vi "函数类型3测试.vi"() -> ()   [LabVIEW 2010]
uses:
  全局量/试验配置信息.vi
panel:
  out "合格？":bool[](array[boolean])
  in  "第几组数据":i32
  in  "同步_A2":i32
  in  "同步_A1":i32
  in  "数组_输入值":enum16{"0", "1"}[](array[ring])
  in  "数组_选择?":bool[](array[boolean])
  in  "btn_置1_5":bool
  in  "btn_置1_4":bool
  in  "btn_置1_3":bool
  in  "btn_置1_2":bool
  in  "btn_全选_5":bool
  in  "btn_全选_4":bool
  in  "btn_全选_3":bool
  in  "btn_全选_2":bool
  in  "btn_置1_1":bool
  in  "btn_全选_1":bool
  in  "CAN端口":u16
  out "light_80":bool
  out "light_79":bool
  out "light_78":bool
  out "light_77":bool
  out "light_76":bool
  out "light_75":bool
  out "light_74":bool
  out "light_73":bool
  out "light_72":bool
  out "light_71":bool
  out "light_70":bool
  out "light_69":bool
  out "light_68":bool
  out "light_67":bool
  out "light_66":bool
  out "light_65":bool
  in  "输入值_73":enum16{"0", "1"}(ring)
  in  "输入值_80":enum16{"0", "1"}(ring)
  in  "输入值_79":enum16{"0", "1"}(ring)
  in  "输入值_78":enum16{"0", "1"}(ring)
  in  "输入值_77":enum16{"0", "1"}(ring)
  in  "输入值_76":enum16{"0", "1"}(ring)
  in  "输入值_75":enum16{"0", "1"}(ring)
  in  "输入值_74":enum16{"0", "1"}(ring)
  in  "输入值_65":enum16{"0", "1"}(ring)
  in  "输入值_72":enum16{"0", "1"}(ring)
  in  "输入值_71":enum16{"0", "1"}(ring)
  in  "输入值_70":enum16{"0", "1"}(ring)
  in  "输入值_69":enum16{"0", "1"}(ring)
  in  "输入值_68":enum16{"0", "1"}(ring)
  in  "输入值_67":enum16{"0", "1"}(ring)
  in  "输入值_66":enum16{"0", "1"}(ring)
  in  "单选_第73路":bool
  in  "单选_第80路":bool
  in  "单选_第79路":bool
  in  "单选_第78路":bool
  in  "单选_第77路":bool
  in  "单选_第76路":bool
  in  "单选_第75路":bool
  in  "单选_第74路":bool
  in  "单选_第65路":bool
  in  "单选_第72路":bool
  in  "单选_第71路":bool
  in  "单选_第70路":bool
  in  "单选_第69路":bool
  in  "单选_第68路":bool
  in  "单选_第67路":bool
  in  "单选_第66路":bool
  out "light_64":bool
  out "light_63":bool
  out "light_62":bool
  out "light_61":bool
  out "light_60":bool
  out "light_59":bool
  out "light_58":bool
  out "light_57":bool
  out "light_56":bool
  out "light_55":bool
  out "light_54":bool
  out "light_53":bool
  out "light_52":bool
  out "light_51":bool
  out "light_50":bool
  out "light_49":bool
  in  "输入值_57":enum16{"0", "1"}(ring)
  in  "输入值_64":enum16{"0", "1"}(ring)
  in  "输入值_63":enum16{"0", "1"}(ring)
  in  "输入值_62":enum16{"0", "1"}(ring)
  in  "输入值_61":enum16{"0", "1"}(ring)
  in  "输入值_60":enum16{"0", "1"}(ring)
  in  "输入值_59":enum16{"0", "1"}(ring)
  in  "输入值_58":enum16{"0", "1"}(ring)
  in  "输入值_49":enum16{"0", "1"}(ring)
  in  "输入值_56":enum16{"0", "1"}(ring)
  in  "输入值_55":enum16{"0", "1"}(ring)
  in  "输入值_54":enum16{"0", "1"}(ring)
  in  "输入值_53":enum16{"0", "1"}(ring)
  in  "输入值_52":enum16{"0", "1"}(ring)
  in  "输入值_51":enum16{"0", "1"}(ring)
  in  "输入值_50":enum16{"0", "1"}(ring)
  in  "单选_第57路":bool
  in  "单选_第64路":bool
  in  "单选_第63路":bool
  in  "单选_第62路":bool
  in  "单选_第61路":bool
  in  "单选_第60路":bool
  in  "单选_第59路":bool
  in  "单选_第58路":bool
  in  "单选_第49路":bool
  in  "单选_第56路":bool
  in  "单选_第55路":bool
  in  "单选_第54路":bool
  in  "单选_第53路":bool
  in  "单选_第52路":bool
  in  "单选_第51路":bool
  in  "单选_第50路":bool
  out "light_48":bool
  out "light_47":bool
  out "light_46":bool
  out "light_45":bool
  out "light_44":bool
  out "light_43":bool
  out "light_42":bool
  out "light_41":bool
  out "light_40":bool
  out "light_39":bool
  out "light_38":bool
  out "light_37":bool
  out "light_36":bool
  out "light_35":bool
  out "light_34":bool
  out "light_33":bool
  in  "输入值_41":enum16{"0", "1"}(ring)
  in  "输入值_48":enum16{"0", "1"}(ring)
  in  "输入值_47":enum16{"0", "1"}(ring)
  in  "输入值_46":enum16{"0", "1"}(ring)
  in  "输入值_45":enum16{"0", "1"}(ring)
  in  "输入值_44":enum16{"0", "1"}(ring)
  in  "输入值_43":enum16{"0", "1"}(ring)
  in  "输入值_42":enum16{"0", "1"}(ring)
  in  "输入值_33":enum16{"0", "1"}(ring)
  in  "输入值_40":enum16{"0", "1"}(ring)
  in  "输入值_39":enum16{"0", "1"}(ring)
  in  "输入值_38":enum16{"0", "1"}(ring)
  in  "输入值_37":enum16{"0", "1"}(ring)
  in  "输入值_36":enum16{"0", "1"}(ring)
  in  "输入值_35":enum16{"0", "1"}(ring)
  in  "输入值_34":enum16{"0", "1"}(ring)
  in  "单选_第41路":bool
  in  "单选_第48路":bool
  in  "单选_第47路":bool
  in  "单选_第46路":bool
  in  "单选_第45路":bool
  in  "单选_第44路":bool
  in  "单选_第43路":bool
  in  "单选_第42路":bool
  in  "单选_第33路":bool
  in  "单选_第40路":bool
  in  "单选_第39路":bool
  in  "单选_第38路":bool
  in  "单选_第37路":bool
  in  "单选_第36路":bool
  in  "单选_第35路":bool
  in  "单选_第34路":bool
  out "light_32":bool
  out "light_31":bool
  out "light_30":bool
  out "light_29":bool
  out "light_28":bool
  out "light_27":bool
  out "light_26":bool
  out "light_25":bool
  out "light_24":bool
  out "light_23":bool
  out "light_22":bool
  out "light_21":bool
  out "light_20":bool
  out "light_19":bool
  out "light_18":bool
  out "light_17":bool
  in  "输入值_25":enum16{"0", "1"}(ring)
  in  "输入值_32":enum16{"0", "1"}(ring)
  in  "输入值_31":enum16{"0", "1"}(ring)
  in  "输入值_30":enum16{"0", "1"}(ring)
  in  "输入值_29":enum16{"0", "1"}(ring)
  in  "输入值_28":enum16{"0", "1"}(ring)
  in  "输入值_27":enum16{"0", "1"}(ring)
  in  "输入值_26":enum16{"0", "1"}(ring)
  in  "输入值_17":enum16{"0", "1"}(ring)
  in  "输入值_24":enum16{"0", "1"}(ring)
  in  "输入值_23":enum16{"0", "1"}(ring)
  in  "输入值_22":enum16{"0", "1"}(ring)
  in  "输入值_21":enum16{"0", "1"}(ring)
  in  "输入值_20":enum16{"0", "1"}(ring)
  in  "输入值_19":enum16{"0", "1"}(ring)
  in  "输入值_18":enum16{"0", "1"}(ring)
  in  "单选_第25路":bool
  in  "单选_第32路":bool
  in  "单选_第31路":bool
  in  "单选_第30路":bool
  in  "单选_第29路":bool
  in  "单选_第28路":bool
  in  "单选_第27路":bool
  in  "单选_第26路":bool
  in  "单选_第17路":bool
  in  "单选_第24路":bool
  in  "单选_第23路":bool
  in  "单选_第22路":bool
  in  "单选_第21路":bool
  in  "单选_第20路":bool
  in  "单选_第19路":bool
  in  "单选_第18路":bool
  in  "D_IN_5":string[][](table) caption="表格"
  in  "D_IN_4":string[][](table) caption="表格"
  in  "D_IN_3":string[][](table) caption="表格"
  in  "D_IN_2":string[][](table) caption="表格"
  out "light_16":bool
  out "light_15":bool
  out "light_14":bool
  out "light_13":bool
  out "light_12":bool
  out "light_11":bool
  out "light_10":bool
  out "light_9":bool
  out "light_8":bool
  out "light_7":bool
  out "light_6":bool
  out "light_5":bool
  out "light_4":bool
  out "light_3":bool
  out "light_2":bool
  out "light_1":bool
  in  "输入值_9":enum16{"0", "1"}(ring)
  in  "输入值_16":enum16{"0", "1"}(ring)
  in  "输入值_15":enum16{"0", "1"}(ring)
  in  "输入值_14":enum16{"0", "1"}(ring)
  in  "输入值_13":enum16{"0", "1"}(ring)
  in  "输入值_12":enum16{"0", "1"}(ring)
  in  "输入值_11":enum16{"0", "1"}(ring)
  in  "输入值_10":enum16{"0", "1"}(ring)
  in  "输入值_1":enum16{"0", "1"}(ring)
  in  "输入值_8":enum16{"0", "1"}(ring)
  in  "输入值_7":enum16{"0", "1"}(ring)
  in  "输入值_6":enum16{"0", "1"}(ring)
  in  "输入值_5":enum16{"0", "1"}(ring)
  in  "输入值_4":enum16{"0", "1"}(ring)
  in  "输入值_3":enum16{"0", "1"}(ring)
  in  "输入值_2":enum16{"0", "1"}(ring)
  in  "单选_第9路":bool
  in  "单选_第16路":bool
  in  "单选_第15路":bool
  in  "单选_第14路":bool
  in  "单选_第13路":bool
  in  "单选_第12路":bool
  in  "单选_第11路":bool
  in  "单选_第10路":bool
  in  "单选_第1路":bool
  in  "单选_第8路":bool
  in  "单选_第7路":bool
  in  "单选_第6路":bool
  in  "单选_第5路":bool
  in  "单选_第4路":bool
  in  "单选_第3路":bool
  in  "单选_第2路":bool
  in  "D_IN_1":string[][](table) caption="表格"
  out "关闭？":bool
  out "测试结论":string
  in  "btn_置0":bool
  in  "btn_置1":bool
  in  "btn_反选":bool
  in  "btn_全选":bool
  in  "btn_关闭":bool
  in  "btn_开始试验":bool
  # "第一组数字量测试"
  # "第二组数字量测试"
  # "第三组数字量测试"
  # "第四组数字量测试"
  # "第五组数字量测试"
  # "测试结论："
  # "80"
  # "80"
  # "80"
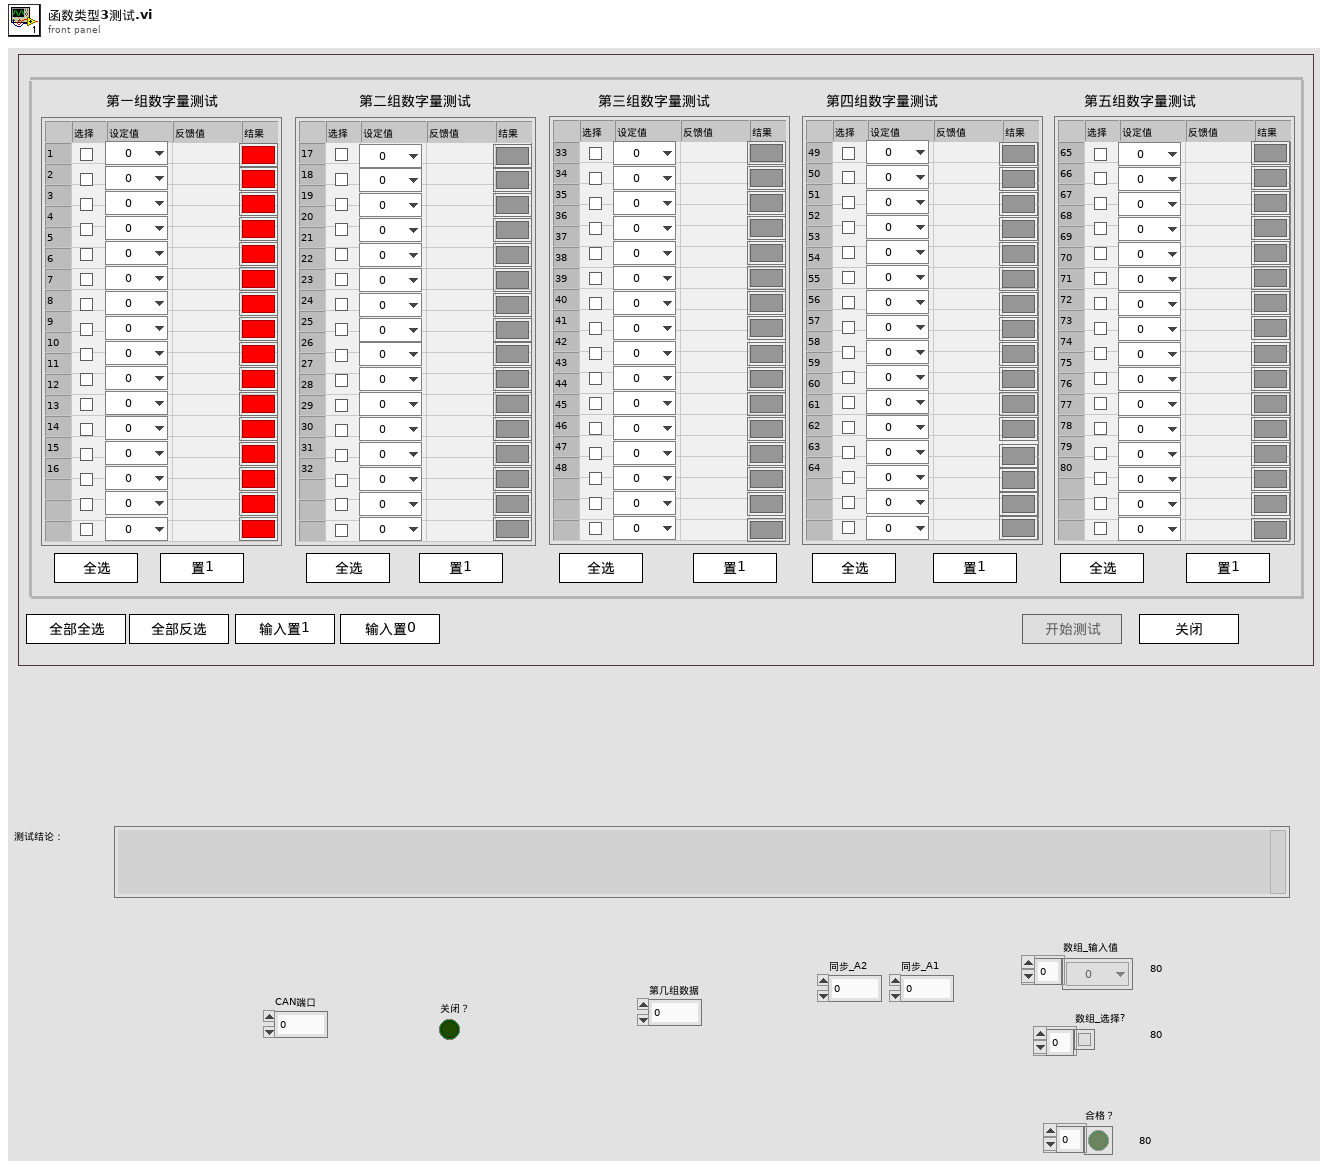
[diagram p1: front panel]
types:
  T1 = enum8{"Enabled", "Disabled", "Disabled and Grayed Out"}
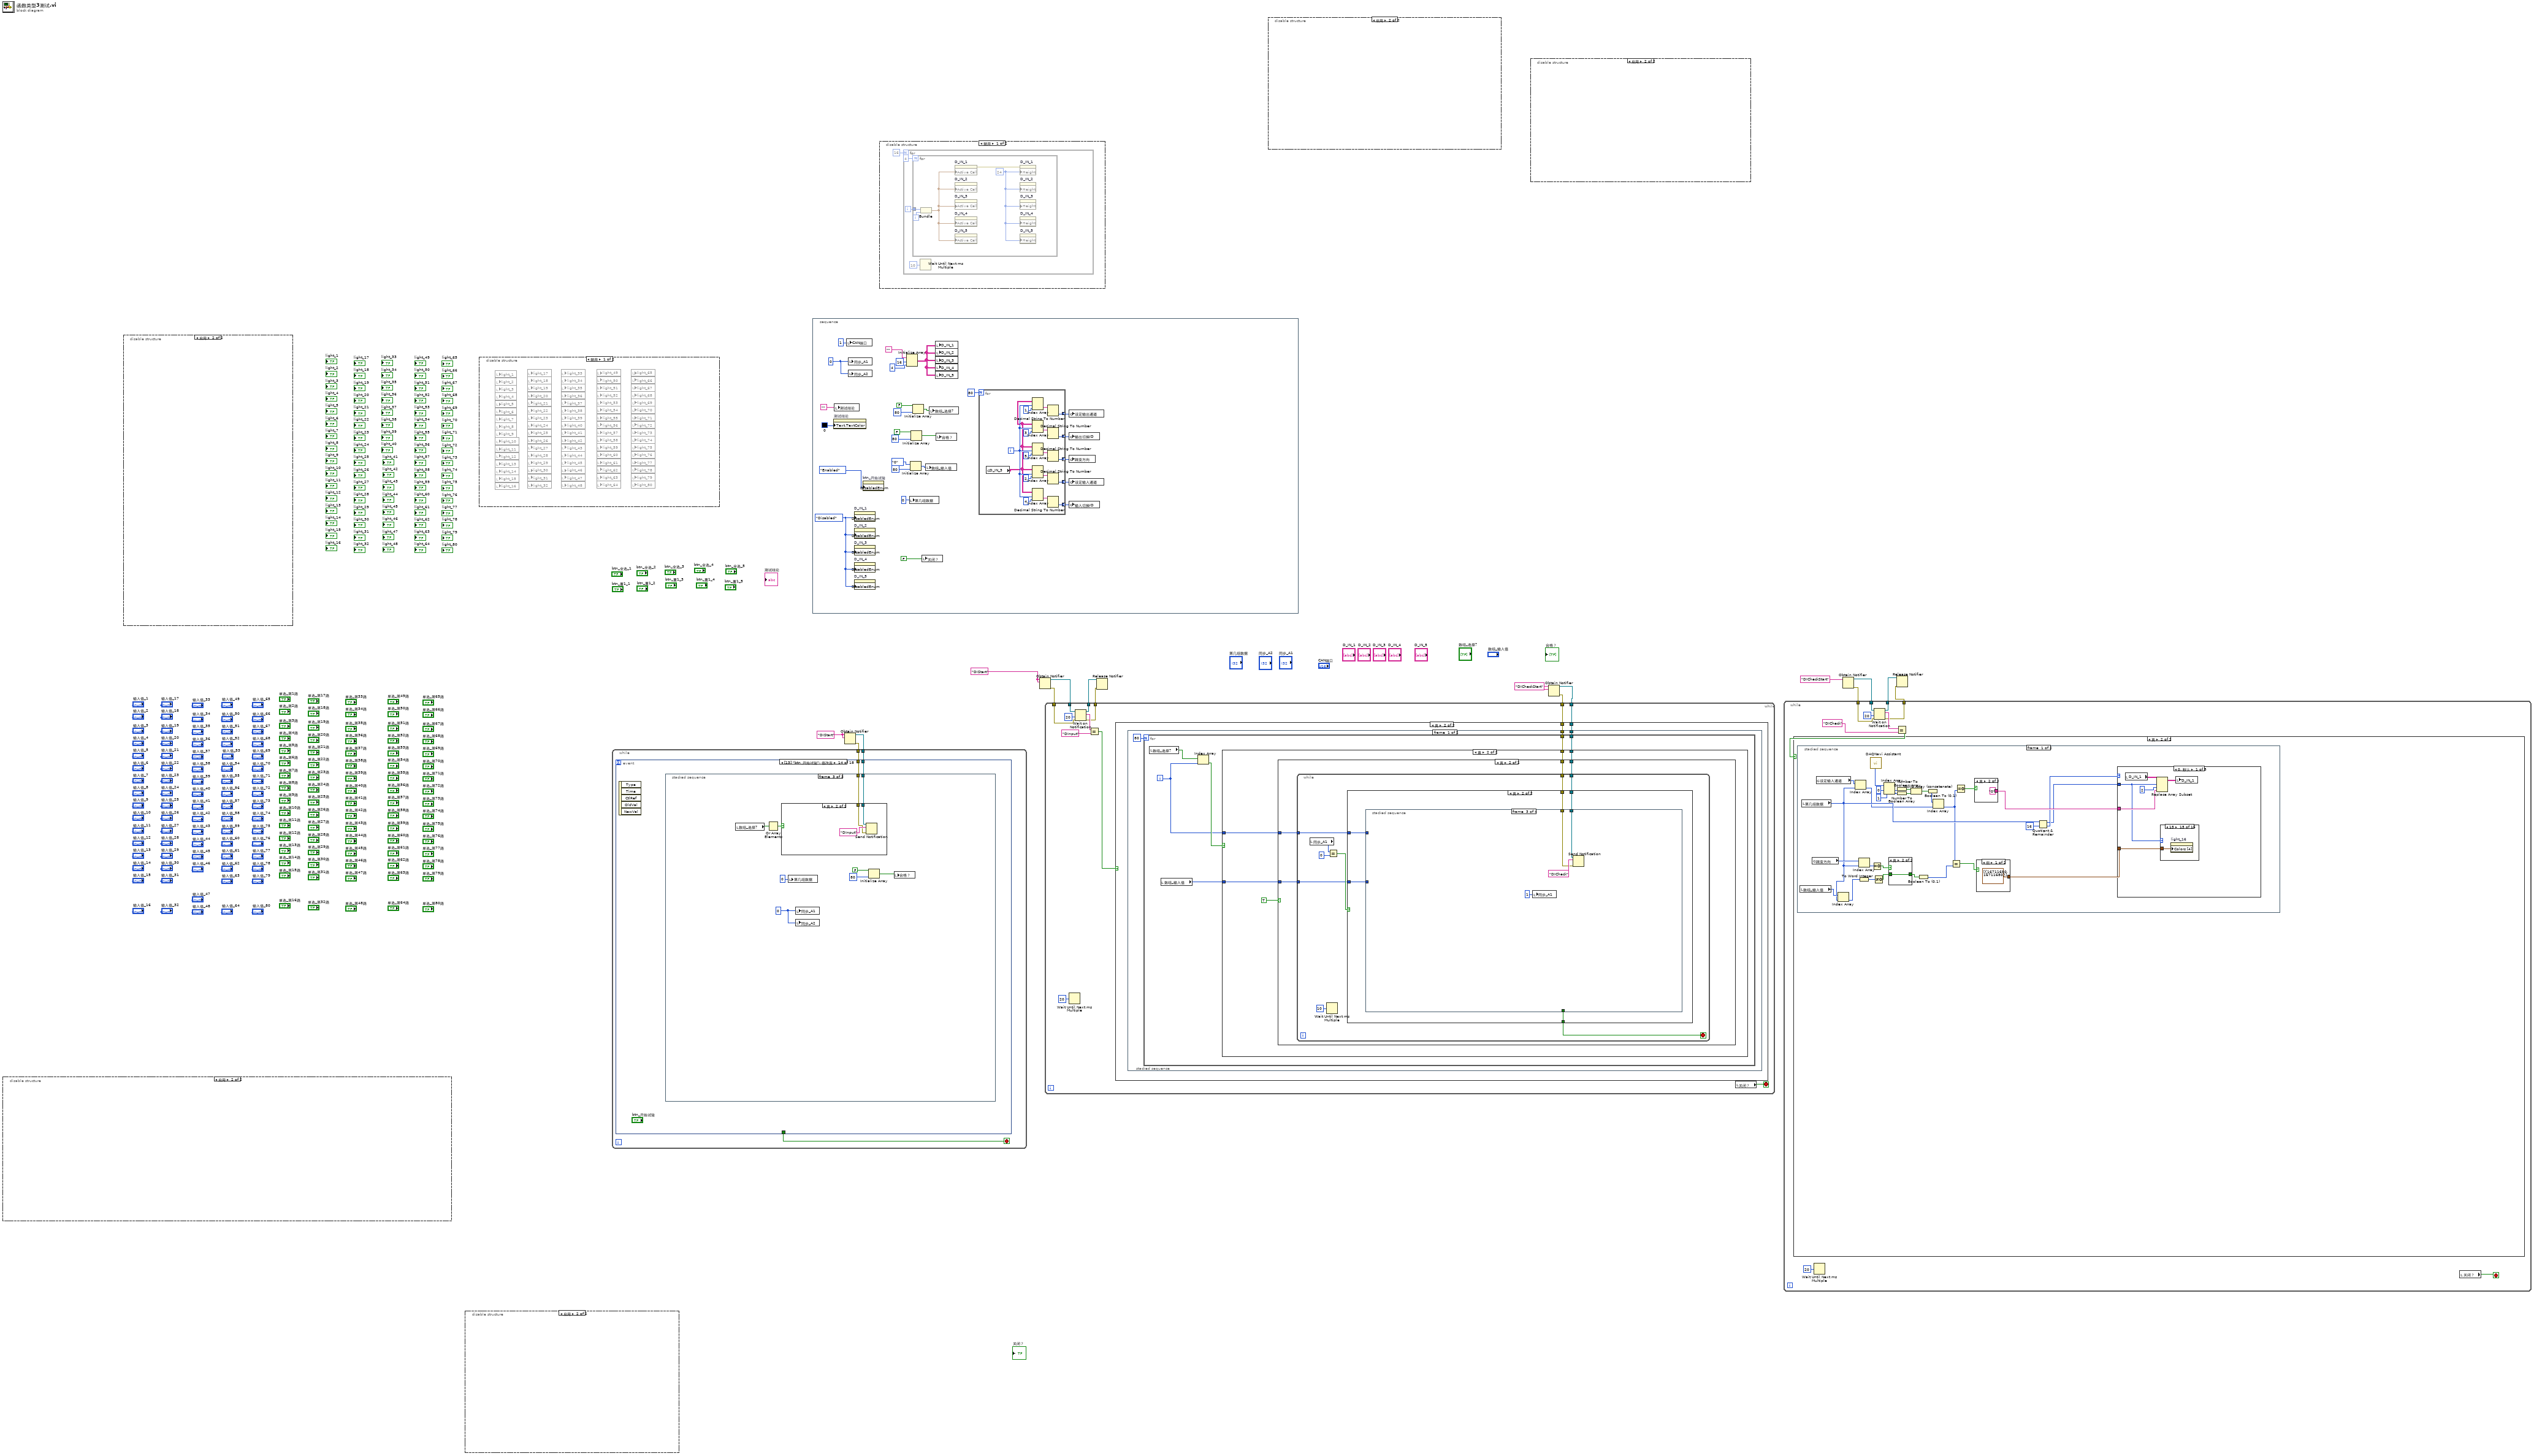
[diagram p0: block diagram]
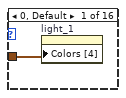
[diagram p4: hidden frame]
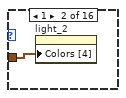
[diagram p5: hidden frame]
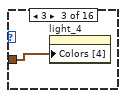
[diagram p6: hidden frame]
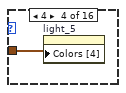
[diagram p7: hidden frame]
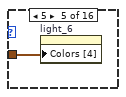
[diagram p8: hidden frame]
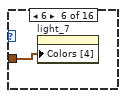
[diagram p9: hidden frame]
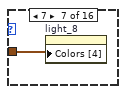
[diagram p10: hidden frame]
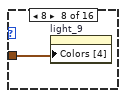
[diagram p11: hidden frame]
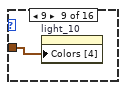
[diagram p12: hidden frame]
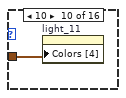
[diagram p13: hidden frame]
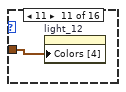
[diagram p14: hidden frame]
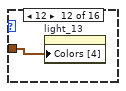
[diagram p15: hidden frame]
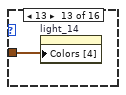
[diagram p16: hidden frame]
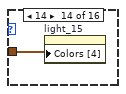
[diagram p17: hidden frame]
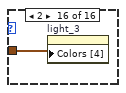
[diagram p18: hidden frame]
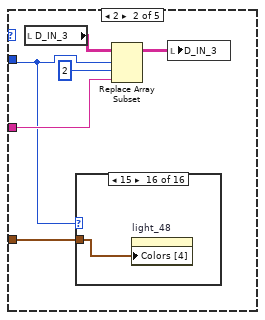
[diagram p19: hidden frame]
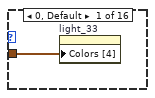
[diagram p20: hidden frame]
diagram:
  w4 = "DICheckStart" ("名称（未命名）")
  w6 = "DIStart" ("名称（未命名）")
  w7 = "DICheckStart" ("名称（未命名）")
  w8 = "DIStart" ("名称（未命名）")
  n1 = disable-structure shown="启用" {
    frame Disabled {
      n2 = local read "单选_第1路"() -> ()  [unwired: 1 in]
      n3 = local read "单选_第2路"() -> ()  [unwired: 1 in]
      n4 = local read "单选_第3路"() -> ()  [unwired: 1 in]
      n5 = local read "单选_第4路"() -> ()  [unwired: 1 in]
      n6 = local read "单选_第5路"() -> ()  [unwired: 1 in]
      n7 = local read "单选_第6路"() -> ()  [unwired: 1 in]
      n8 = local read "单选_第7路"() -> ()  [unwired: 1 in]
      n9 = local read "单选_第8路"() -> ()  [unwired: 1 in]
      n10 = local read "单选_第9路"() -> ()  [unwired: 1 in]
      n11 = local read "单选_第10路"() -> ()  [unwired: 1 in]
      n12 = local read "单选_第11路"() -> ()  [unwired: 1 in]
      n13 = local read "单选_第12路"() -> ()  [unwired: 1 in]
      n14 = local read "单选_第13路"() -> ()  [unwired: 1 in]
      n15 = local read "单选_第14路"() -> ()  [unwired: 1 in]
      n16 = local read "单选_第15路"() -> ()  [unwired: 1 in]
      n17 = local read "单选_第16路"() -> ()  [unwired: 1 in]
      n18 = local read "单选_第17路"() -> ()  [unwired: 1 in]
      n19 = local read "单选_第18路"() -> ()  [unwired: 1 in]
      n20 = local read "单选_第19路"() -> ()  [unwired: 1 in]
      n21 = local read "单选_第20路"() -> ()  [unwired: 1 in]
      n22 = local read "单选_第21路"() -> ()  [unwired: 1 in]
      n23 = local read "单选_第22路"() -> ()  [unwired: 1 in]
      n24 = local read "单选_第23路"() -> ()  [unwired: 1 in]
      n25 = local read "单选_第24路"() -> ()  [unwired: 1 in]
      n26 = local read "单选_第25路"() -> ()  [unwired: 1 in]
      n27 = local read "单选_第26路"() -> ()  [unwired: 1 in]
      n28 = local read "单选_第27路"() -> ()  [unwired: 1 in]
      n29 = local read "单选_第28路"() -> ()  [unwired: 1 in]
      n30 = local read "单选_第29路"() -> ()  [unwired: 1 in]
      n31 = local read "单选_第30路"() -> ()  [unwired: 1 in]
      n32 = local read "单选_第31路"() -> ()  [unwired: 1 in]
      n33 = local read "单选_第32路"() -> ()  [unwired: 1 in]
      n34 = local read "单选_第33路"() -> ()  [unwired: 1 in]
      n35 = local read "单选_第34路"() -> ()  [unwired: 1 in]
      n36 = local read "单选_第35路"() -> ()  [unwired: 1 in]
      n37 = local read "单选_第36路"() -> ()  [unwired: 1 in]
      n38 = local read "单选_第37路"() -> ()  [unwired: 1 in]
      n39 = local read "单选_第38路"() -> ()  [unwired: 1 in]
      n40 = local read "单选_第39路"() -> ()  [unwired: 1 in]
      n41 = local read "单选_第40路"() -> ()  [unwired: 1 in]
      n42 = local read "单选_第41路"() -> ()  [unwired: 1 in]
      n43 = local read "单选_第42路"() -> ()  [unwired: 1 in]
      n44 = local read "单选_第43路"() -> ()  [unwired: 1 in]
      n45 = local read "单选_第44路"() -> ()  [unwired: 1 in]
      n46 = local read "单选_第45路"() -> ()  [unwired: 1 in]
      n47 = local read "单选_第46路"() -> ()  [unwired: 1 in]
      n48 = local read "单选_第47路"() -> ()  [unwired: 1 in]
      n49 = local read "单选_第48路"() -> ()  [unwired: 1 in]
      n50 = local read "单选_第49路"() -> ()  [unwired: 1 in]
      n51 = local read "单选_第50路"() -> ()  [unwired: 1 in]
      n52 = local read "单选_第51路"() -> ()  [unwired: 1 in]
      n53 = local read "单选_第52路"() -> ()  [unwired: 1 in]
      n54 = local read "单选_第53路"() -> ()  [unwired: 1 in]
      n55 = local read "单选_第54路"() -> ()  [unwired: 1 in]
      n56 = local read "单选_第55路"() -> ()  [unwired: 1 in]
      n57 = local read "单选_第56路"() -> ()  [unwired: 1 in]
      n58 = local read "单选_第57路"() -> ()  [unwired: 1 in]
      n59 = local read "单选_第58路"() -> ()  [unwired: 1 in]
      n60 = local read "单选_第59路"() -> ()  [unwired: 1 in]
      n61 = local read "单选_第60路"() -> ()  [unwired: 1 in]
      n62 = local read "单选_第61路"() -> ()  [unwired: 1 in]
      n63 = local read "单选_第62路"() -> ()  [unwired: 1 in]
      n64 = local read "单选_第63路"() -> ()  [unwired: 1 in]
      n65 = local read "单选_第64路"() -> ()  [unwired: 1 in]
      n66 = local read "单选_第71路"() -> ()  [unwired: 1 in]
      n67 = local read "单选_第79路"() -> ()  [unwired: 1 in]
      n68 = local read "单选_第65路"() -> ()  [unwired: 1 in]
      n69 = local read "单选_第66路"() -> ()  [unwired: 1 in]
      n70 = local read "单选_第67路"() -> ()  [unwired: 1 in]
      n71 = local read "单选_第68路"() -> ()  [unwired: 1 in]
      n72 = local read "单选_第69路"() -> ()  [unwired: 1 in]
      n73 = local read "单选_第70路"() -> ()  [unwired: 1 in]
      n74 = local read "单选_第72路"() -> ()  [unwired: 1 in]
      n75 = local read "单选_第73路"() -> ()  [unwired: 1 in]
      n76 = local read "单选_第74路"() -> ()  [unwired: 1 in]
      n77 = local read "单选_第75路"() -> ()  [unwired: 1 in]
      n78 = local read "单选_第76路"() -> ()  [unwired: 1 in]
      n79 = local read "单选_第77路"() -> ()  [unwired: 1 in]
      n80 = local read "单选_第78路"() -> ()  [unwired: 1 in]
      n81 = local read "单选_第80路"() -> ()  [unwired: 1 in]
      n82 = local read "输入值_1"() -> ()  [unwired: 1 in]
      n83 = local read "输入值_2"() -> ()  [unwired: 1 in]
      n84 = local read "输入值_3"() -> ()  [unwired: 1 in]
      n85 = local read "输入值_4"() -> ()  [unwired: 1 in]
      n86 = local read "输入值_5"() -> ()  [unwired: 1 in]
      n87 = local read "输入值_6"() -> ()  [unwired: 1 in]
      n88 = local read "输入值_7"() -> ()  [unwired: 1 in]
      n89 = local read "输入值_8"() -> ()  [unwired: 1 in]
      n90 = local read "输入值_9"() -> ()  [unwired: 1 in]
      n91 = local read "输入值_10"() -> ()  [unwired: 1 in]
      n92 = local read "输入值_11"() -> ()  [unwired: 1 in]
      n93 = local read "输入值_12"() -> ()  [unwired: 1 in]
      n94 = local read "输入值_13"() -> ()  [unwired: 1 in]
      n95 = local read "输入值_14"() -> ()  [unwired: 1 in]
      n96 = local read "输入值_15"() -> ()  [unwired: 1 in]
      n97 = local read "输入值_16"() -> ()  [unwired: 1 in]
      n98 = local read "输入值_17"() -> ()  [unwired: 1 in]
      n99 = local read "输入值_18"() -> ()  [unwired: 1 in]
      n100 = local read "输入值_19"() -> ()  [unwired: 1 in]
      n101 = local read "输入值_20"() -> ()  [unwired: 1 in]
      n102 = local read "输入值_21"() -> ()  [unwired: 1 in]
      n103 = local read "输入值_22"() -> ()  [unwired: 1 in]
      n104 = local read "输入值_23"() -> ()  [unwired: 1 in]
      n105 = local read "输入值_24"() -> ()  [unwired: 1 in]
      n106 = local read "输入值_25"() -> ()  [unwired: 1 in]
      n107 = local read "输入值_26"() -> ()  [unwired: 1 in]
      n108 = local read "输入值_27"() -> ()  [unwired: 1 in]
      n109 = local read "输入值_28"() -> ()  [unwired: 1 in]
      n110 = local read "输入值_29"() -> ()  [unwired: 1 in]
      n111 = local read "输入值_30"() -> ()  [unwired: 1 in]
      n112 = local read "输入值_31"() -> ()  [unwired: 1 in]
      n113 = local read "输入值_32"() -> ()  [unwired: 1 in]
      n114 = local read "输入值_33"() -> ()  [unwired: 1 in]
      n115 = local read "输入值_34"() -> ()  [unwired: 1 in]
      n116 = local read "输入值_35"() -> ()  [unwired: 1 in]
      n117 = local read "输入值_36"() -> ()  [unwired: 1 in]
      n118 = local read "输入值_37"() -> ()  [unwired: 1 in]
      n119 = local read "输入值_38"() -> ()  [unwired: 1 in]
      n120 = local read "输入值_39"() -> ()  [unwired: 1 in]
      n121 = local read "输入值_40"() -> ()  [unwired: 1 in]
      n122 = local read "输入值_41"() -> ()  [unwired: 1 in]
      n123 = local read "输入值_42"() -> ()  [unwired: 1 in]
      n124 = local read "输入值_43"() -> ()  [unwired: 1 in]
      n125 = local read "输入值_44"() -> ()  [unwired: 1 in]
      n126 = local read "输入值_45"() -> ()  [unwired: 1 in]
      n127 = local read "输入值_46"() -> ()  [unwired: 1 in]
      n128 = local read "输入值_47"() -> ()  [unwired: 1 in]
      n129 = local read "输入值_48"() -> ()  [unwired: 1 in]
      n130 = local read "输入值_49"() -> ()  [unwired: 1 in]
      n131 = local read "输入值_50"() -> ()  [unwired: 1 in]
      n132 = local read "输入值_51"() -> ()  [unwired: 1 in]
      n133 = local read "输入值_52"() -> ()  [unwired: 1 in]
      n134 = local read "输入值_53"() -> ()  [unwired: 1 in]
      n135 = local read "输入值_54"() -> ()  [unwired: 1 in]
      n136 = local read "输入值_55"() -> ()  [unwired: 1 in]
      n137 = local read "输入值_56"() -> ()  [unwired: 1 in]
      n138 = local read "输入值_57"() -> ()  [unwired: 1 in]
      n139 = local read "输入值_58"() -> ()  [unwired: 1 in]
      n140 = local read "输入值_59"() -> ()  [unwired: 1 in]
      n141 = local read "输入值_60"() -> ()  [unwired: 1 in]
      n142 = local read "输入值_61"() -> ()  [unwired: 1 in]
      n143 = local read "输入值_62"() -> ()  [unwired: 1 in]
      n144 = local read "输入值_63"() -> ()  [unwired: 1 in]
      n145 = local read "输入值_64"() -> ()  [unwired: 1 in]
      n146 = local read "输入值_65"() -> ()  [unwired: 1 in]
      n147 = local read "输入值_66"() -> ()  [unwired: 1 in]
      n148 = local read "输入值_67"() -> ()  [unwired: 1 in]
      n149 = local read "输入值_68"() -> ()  [unwired: 1 in]
      n150 = local read "输入值_69"() -> ()  [unwired: 1 in]
      n151 = local read "输入值_70"() -> ()  [unwired: 1 in]
      n152 = local read "输入值_71"() -> ()  [unwired: 1 in]
      n153 = local read "输入值_72"() -> ()  [unwired: 1 in]
      n154 = local read "输入值_73"() -> ()  [unwired: 1 in]
      n155 = local read "输入值_74"() -> ()  [unwired: 1 in]
      n156 = local read "输入值_75"() -> ()  [unwired: 1 in]
      n157 = local read "输入值_76"() -> ()  [unwired: 1 in]
      n158 = local read "输入值_77"() -> ()  [unwired: 1 in]
      n159 = local read "输入值_78"() -> ()  [unwired: 1 in]
      n160 = local read "输入值_79"() -> ()  [unwired: 1 in]
      n161 = local read "输入值_80"() -> ()  [unwired: 1 in]
    }
    frame Enabled {
    }
  }
  n162 = disable-structure shown="启用" {
    frame Disabled {
      n163 = property on="light_1" class="Bool (严格)" props=["Colors [4]"]() -> ()  [unwired: 3 in, 2 out]
      n164 = property on="light_2" class="Bool (严格)" props=["Colors [4]"]() -> ()  [unwired: 3 in, 2 out]
      n165 = property on="light_3" class="Bool (严格)" props=["Colors [4]"]() -> ()  [unwired: 3 in, 2 out]
      n166 = property on="light_4" class="Bool (严格)" props=["Colors [4]"]() -> ()  [unwired: 3 in, 2 out]
      n167 = property on="light_5" class="Bool (严格)" props=["Colors [4]"]() -> ()  [unwired: 3 in, 2 out]
      n168 = property on="light_6" class="Bool (严格)" props=["Colors [4]"]() -> ()  [unwired: 3 in, 2 out]
      n169 = property on="light_7" class="Bool (严格)" props=["Colors [4]"]() -> ()  [unwired: 3 in, 2 out]
      n170 = property on="light_8" class="Bool (严格)" props=["Colors [4]"]() -> ()  [unwired: 3 in, 2 out]
      n171 = property on="light_9" class="Bool (严格)" props=["Colors [4]"]() -> ()  [unwired: 3 in, 2 out]
      n172 = property on="light_10" class="Bool (严格)" props=["Colors [4]"]() -> ()  [unwired: 3 in, 2 out]
      n173 = property on="light_11" class="Bool (严格)" props=["Colors [4]"]() -> ()  [unwired: 3 in, 2 out]
      n174 = property on="light_12" class="Bool (严格)" props=["Colors [4]"]() -> ()  [unwired: 3 in, 2 out]
      n175 = property on="light_13" class="Bool (严格)" props=["Colors [4]"]() -> ()  [unwired: 3 in, 2 out]
      n176 = property on="light_14" class="Bool (严格)" props=["Colors [4]"]() -> ()  [unwired: 3 in, 2 out]
      n177 = property on="light_15" class="Bool (严格)" props=["Colors [4]"]() -> ()  [unwired: 3 in, 2 out]
      n178 = property on="light_16" class="Bool (严格)" props=["Colors [4]"]() -> ()  [unwired: 3 in, 2 out]
      n179 = property on="light_17" class="Bool (严格)" props=["Colors [4]"]() -> ()  [unwired: 3 in, 2 out]
      n180 = property on="light_18" class="Bool (严格)" props=["Colors [4]"]() -> ()  [unwired: 3 in, 2 out]
      n181 = property on="light_19" class="Bool (严格)" props=["Colors [4]"]() -> ()  [unwired: 3 in, 2 out]
      n182 = property on="light_20" class="Bool (严格)" props=["Colors [4]"]() -> ()  [unwired: 3 in, 2 out]
      n183 = property on="light_21" class="Bool (严格)" props=["Colors [4]"]() -> ()  [unwired: 3 in, 2 out]
      n184 = property on="light_22" class="Bool (严格)" props=["Colors [4]"]() -> ()  [unwired: 3 in, 2 out]
      n185 = property on="light_23" class="Bool (严格)" props=["Colors [4]"]() -> ()  [unwired: 3 in, 2 out]
      n186 = property on="light_24" class="Bool (严格)" props=["Colors [4]"]() -> ()  [unwired: 3 in, 2 out]
      n187 = property on="light_25" class="Bool (严格)" props=["Colors [4]"]() -> ()  [unwired: 3 in, 2 out]
      n188 = property on="light_26" class="Bool (严格)" props=["Colors [4]"]() -> ()  [unwired: 3 in, 2 out]
      n189 = property on="light_27" class="Bool (严格)" props=["Colors [4]"]() -> ()  [unwired: 3 in, 2 out]
      n190 = property on="light_28" class="Bool (严格)" props=["Colors [4]"]() -> ()  [unwired: 3 in, 2 out]
      n191 = property on="light_29" class="Bool (严格)" props=["Colors [4]"]() -> ()  [unwired: 3 in, 2 out]
      n192 = property on="light_30" class="Bool (严格)" props=["Colors [4]"]() -> ()  [unwired: 3 in, 2 out]
      n193 = property on="light_31" class="Bool (严格)" props=["Colors [4]"]() -> ()  [unwired: 3 in, 2 out]
      n194 = property on="light_32" class="Bool (严格)" props=["Colors [4]"]() -> ()  [unwired: 3 in, 2 out]
      n195 = property on="light_33" class="Bool (严格)" props=["Colors [4]"]() -> ()  [unwired: 3 in, 2 out]
      n196 = property on="light_34" class="Bool (严格)" props=["Colors [4]"]() -> ()  [unwired: 3 in, 2 out]
      n197 = property on="light_35" class="Bool (严格)" props=["Colors [4]"]() -> ()  [unwired: 3 in, 2 out]
      n198 = property on="light_36" class="Bool (严格)" props=["Colors [4]"]() -> ()  [unwired: 3 in, 2 out]
      n199 = property on="light_37" class="Bool (严格)" props=["Colors [4]"]() -> ()  [unwired: 3 in, 2 out]
      n200 = property on="light_38" class="Bool (严格)" props=["Colors [4]"]() -> ()  [unwired: 3 in, 2 out]
      n201 = property on="light_39" class="Bool (严格)" props=["Colors [4]"]() -> ()  [unwired: 3 in, 2 out]
      n202 = property on="light_40" class="Bool (严格)" props=["Colors [4]"]() -> ()  [unwired: 3 in, 2 out]
      n203 = property on="light_41" class="Bool (严格)" props=["Colors [4]"]() -> ()  [unwired: 3 in, 2 out]
      n204 = property on="light_42" class="Bool (严格)" props=["Colors [4]"]() -> ()  [unwired: 3 in, 2 out]
      n205 = property on="light_43" class="Bool (严格)" props=["Colors [4]"]() -> ()  [unwired: 3 in, 2 out]
      n206 = property on="light_44" class="Bool (严格)" props=["Colors [4]"]() -> ()  [unwired: 3 in, 2 out]
      n207 = property on="light_45" class="Bool (严格)" props=["Colors [4]"]() -> ()  [unwired: 3 in, 2 out]
      n208 = property on="light_46" class="Bool (严格)" props=["Colors [4]"]() -> ()  [unwired: 3 in, 2 out]
      n209 = property on="light_47" class="Bool (严格)" props=["Colors [4]"]() -> ()  [unwired: 3 in, 2 out]
      n210 = property on="light_48" class="Bool (严格)" props=["Colors [4]"]() -> ()  [unwired: 3 in, 2 out]
      n211 = property on="light_49" class="Bool (严格)" props=["Colors [4]"]() -> ()  [unwired: 3 in, 2 out]
      n212 = property on="light_50" class="Bool (严格)" props=["Colors [4]"]() -> ()  [unwired: 3 in, 2 out]
      n213 = property on="light_51" class="Bool (严格)" props=["Colors [4]"]() -> ()  [unwired: 3 in, 2 out]
      n214 = property on="light_52" class="Bool (严格)" props=["Colors [4]"]() -> ()  [unwired: 3 in, 2 out]
      n215 = property on="light_53" class="Bool (严格)" props=["Colors [4]"]() -> ()  [unwired: 3 in, 2 out]
      n216 = property on="light_54" class="Bool (严格)" props=["Colors [4]"]() -> ()  [unwired: 3 in, 2 out]
      n217 = property on="light_55" class="Bool (严格)" props=["Colors [4]"]() -> ()  [unwired: 3 in, 2 out]
      n218 = property on="light_56" class="Bool (严格)" props=["Colors [4]"]() -> ()  [unwired: 3 in, 2 out]
      n219 = property on="light_57" class="Bool (严格)" props=["Colors [4]"]() -> ()  [unwired: 3 in, 2 out]
      n220 = property on="light_58" class="Bool (严格)" props=["Colors [4]"]() -> ()  [unwired: 3 in, 2 out]
      n221 = property on="light_59" class="Bool (严格)" props=["Colors [4]"]() -> ()  [unwired: 3 in, 2 out]
      n222 = property on="light_60" class="Bool (严格)" props=["Colors [4]"]() -> ()  [unwired: 3 in, 2 out]
      n223 = property on="light_61" class="Bool (严格)" props=["Colors [4]"]() -> ()  [unwired: 3 in, 2 out]
      n224 = property on="light_62" class="Bool (严格)" props=["Colors [4]"]() -> ()  [unwired: 3 in, 2 out]
      n225 = property on="light_63" class="Bool (严格)" props=["Colors [4]"]() -> ()  [unwired: 3 in, 2 out]
      n226 = property on="light_64" class="Bool (严格)" props=["Colors [4]"]() -> ()  [unwired: 3 in, 2 out]
      n227 = property on="light_65" class="Bool (严格)" props=["Colors [4]"]() -> ()  [unwired: 3 in, 2 out]
      n228 = property on="light_66" class="Bool (严格)" props=["Colors [4]"]() -> ()  [unwired: 3 in, 2 out]
      n229 = property on="light_67" class="Bool (严格)" props=["Colors [4]"]() -> ()  [unwired: 3 in, 2 out]
      n230 = property on="light_68" class="Bool (严格)" props=["Colors [4]"]() -> ()  [unwired: 3 in, 2 out]
      n231 = property on="light_69" class="Bool (严格)" props=["Colors [4]"]() -> ()  [unwired: 3 in, 2 out]
      n232 = property on="light_70" class="Bool (严格)" props=["Colors [4]"]() -> ()  [unwired: 3 in, 2 out]
      n233 = property on="light_71" class="Bool (严格)" props=["Colors [4]"]() -> ()  [unwired: 3 in, 2 out]
      n234 = property on="light_72" class="Bool (严格)" props=["Colors [4]"]() -> ()  [unwired: 3 in, 2 out]
      n235 = property on="light_73" class="Bool (严格)" props=["Colors [4]"]() -> ()  [unwired: 3 in, 2 out]
      n236 = property on="light_74" class="Bool (严格)" props=["Colors [4]"]() -> ()  [unwired: 3 in, 2 out]
      n237 = property on="light_75" class="Bool (严格)" props=["Colors [4]"]() -> ()  [unwired: 3 in, 2 out]
      n238 = property on="light_76" class="Bool (严格)" props=["Colors [4]"]() -> ()  [unwired: 3 in, 2 out]
      n239 = property on="light_77" class="Bool (严格)" props=["Colors [4]"]() -> ()  [unwired: 3 in, 2 out]
      n240 = property on="light_78" class="Bool (严格)" props=["Colors [4]"]() -> ()  [unwired: 3 in, 2 out]
      n241 = property on="light_79" class="Bool (严格)" props=["Colors [4]"]() -> ()  [unwired: 3 in, 2 out]
      n242 = property on="light_80" class="Bool (严格)" props=["Colors [4]"]() -> ()  [unwired: 3 in, 2 out]
    }
    frame Enabled {
    }
  }
  n243 = disable-structure shown="启用" {
    frame Disabled {
      n244 = local read "输入值_1"() -> ()  [unwired: 1 out]
      n245 = local read "输入值_2"() -> ()  [unwired: 1 out]
      n246 = local read "输入值_3"() -> ()  [unwired: 1 out]
      n247 = local read "输入值_4"() -> ()  [unwired: 1 out]
      n248 = local read "输入值_5"() -> ()  [unwired: 1 out]
      n249 = local read "输入值_6"() -> ()  [unwired: 1 out]
      n250 = local read "输入值_7"() -> ()  [unwired: 1 out]
      n251 = local read "输入值_8"() -> ()  [unwired: 1 out]
      n252 = local read "输入值_9"() -> ()  [unwired: 1 out]
      n253 = local read "输入值_10"() -> ()  [unwired: 1 out]
      n254 = local read "输入值_11"() -> ()  [unwired: 1 out]
      n255 = local read "输入值_12"() -> ()  [unwired: 1 out]
      n256 = local read "输入值_13"() -> ()  [unwired: 1 out]
      n257 = local read "输入值_14"() -> ()  [unwired: 1 out]
      n258 = local read "输入值_15"() -> ()  [unwired: 1 out]
      n259 = local read "输入值_16"() -> ()  [unwired: 1 out]
      n260 = local read "输入值_17"() -> ()  [unwired: 1 out]
      n261 = local read "输入值_18"() -> ()  [unwired: 1 out]
      n262 = local read "输入值_19"() -> ()  [unwired: 1 out]
      n263 = local read "输入值_20"() -> ()  [unwired: 1 out]
      n264 = local read "输入值_21"() -> ()  [unwired: 1 out]
      n265 = local read "输入值_22"() -> ()  [unwired: 1 out]
      n266 = local read "输入值_23"() -> ()  [unwired: 1 out]
      n267 = local read "输入值_24"() -> ()  [unwired: 1 out]
      n268 = local read "输入值_25"() -> ()  [unwired: 1 out]
      n269 = local read "输入值_26"() -> ()  [unwired: 1 out]
      n270 = local read "输入值_27"() -> ()  [unwired: 1 out]
      n271 = local read "输入值_28"() -> ()  [unwired: 1 out]
      n272 = local read "输入值_29"() -> ()  [unwired: 1 out]
      n273 = local read "输入值_30"() -> ()  [unwired: 1 out]
      n274 = local read "输入值_31"() -> ()  [unwired: 1 out]
      n275 = local read "输入值_32"() -> ()  [unwired: 1 out]
      n276 = local read "输入值_33"() -> ()  [unwired: 1 out]
      n277 = local read "输入值_34"() -> ()  [unwired: 1 out]
      n278 = local read "输入值_35"() -> ()  [unwired: 1 out]
      n279 = local read "输入值_36"() -> ()  [unwired: 1 out]
      n280 = local read "输入值_37"() -> ()  [unwired: 1 out]
      n281 = local read "输入值_38"() -> ()  [unwired: 1 out]
      n282 = local read "输入值_39"() -> ()  [unwired: 1 out]
      n283 = local read "输入值_40"() -> ()  [unwired: 1 out]
      n284 = local read "输入值_41"() -> ()  [unwired: 1 out]
      n285 = local read "输入值_42"() -> ()  [unwired: 1 out]
      n286 = local read "输入值_43"() -> ()  [unwired: 1 out]
      n287 = local read "输入值_44"() -> ()  [unwired: 1 out]
      n288 = local read "输入值_45"() -> ()  [unwired: 1 out]
      n289 = local read "输入值_46"() -> ()  [unwired: 1 out]
      n290 = local read "输入值_47"() -> ()  [unwired: 1 out]
      n291 = local read "输入值_48"() -> ()  [unwired: 1 out]
      n292 = local read "输入值_49"() -> ()  [unwired: 1 out]
      n293 = local read "输入值_50"() -> ()  [unwired: 1 out]
      n294 = local read "输入值_51"() -> ()  [unwired: 1 out]
      n295 = local read "输入值_52"() -> ()  [unwired: 1 out]
      n296 = local read "输入值_53"() -> ()  [unwired: 1 out]
      n297 = local read "输入值_54"() -> ()  [unwired: 1 out]
      n298 = local read "输入值_55"() -> ()  [unwired: 1 out]
      n299 = local read "输入值_56"() -> ()  [unwired: 1 out]
      n300 = local read "输入值_57"() -> ()  [unwired: 1 out]
      n301 = local read "输入值_58"() -> ()  [unwired: 1 out]
      n302 = local read "输入值_59"() -> ()  [unwired: 1 out]
      n303 = local read "输入值_60"() -> ()  [unwired: 1 out]
      n304 = local read "输入值_61"() -> ()  [unwired: 1 out]
      n305 = local read "输入值_62"() -> ()  [unwired: 1 out]
      n306 = local read "输入值_63"() -> ()  [unwired: 1 out]
      n307 = local read "输入值_64"() -> ()  [unwired: 1 out]
      n308 = local read "输入值_65"() -> ()  [unwired: 1 out]
      n309 = local read "输入值_66"() -> ()  [unwired: 1 out]
      n310 = local read "输入值_67"() -> ()  [unwired: 1 out]
      n311 = local read "输入值_68"() -> ()  [unwired: 1 out]
      n312 = local read "输入值_69"() -> ()  [unwired: 1 out]
      n313 = local read "输入值_70"() -> ()  [unwired: 1 out]
      n314 = local read "输入值_71"() -> ()  [unwired: 1 out]
      n315 = local read "输入值_72"() -> ()  [unwired: 1 out]
      n316 = local read "输入值_73"() -> ()  [unwired: 1 out]
      n317 = local read "输入值_74"() -> ()  [unwired: 1 out]
      n318 = local read "输入值_75"() -> ()  [unwired: 1 out]
      n319 = local read "输入值_76"() -> ()  [unwired: 1 out]
      n320 = local read "输入值_77"() -> ()  [unwired: 1 out]
      n321 = local read "输入值_78"() -> ()  [unwired: 1 out]
      n322 = local read "输入值_79"() -> ()  [unwired: 1 out]
      n323 = local read "输入值_80"() -> ()  [unwired: 1 out]
    }
    frame Enabled {
    }
  }
  n324 = disable-structure shown="禁用" {
    frame Disabled {
      n325 = local read "light_1"() -> ()  [unwired: 1 in]
      n326 = local read "light_2"() -> ()  [unwired: 1 in]
      n327 = local read "light_3"() -> ()  [unwired: 1 in]
      n328 = local read "light_4"() -> ()  [unwired: 1 in]
      n329 = local read "light_5"() -> ()  [unwired: 1 in]
      n330 = local read "light_6"() -> ()  [unwired: 1 in]
      n331 = local read "light_7"() -> ()  [unwired: 1 in]
      n332 = local read "light_8"() -> ()  [unwired: 1 in]
      n333 = local read "light_9"() -> ()  [unwired: 1 in]
      n334 = local read "light_10"() -> ()  [unwired: 1 in]
      n335 = local read "light_11"() -> ()  [unwired: 1 in]
      n336 = local read "light_12"() -> ()  [unwired: 1 in]
      n337 = local read "light_13"() -> ()  [unwired: 1 in]
      n338 = local read "light_14"() -> ()  [unwired: 1 in]
      n339 = local read "light_15"() -> ()  [unwired: 1 in]
      n340 = local read "light_16"() -> ()  [unwired: 1 in]
      n341 = local read "light_17"() -> ()  [unwired: 1 in]
      n342 = local read "light_18"() -> ()  [unwired: 1 in]
      n343 = local read "light_19"() -> ()  [unwired: 1 in]
      n344 = local read "light_20"() -> ()  [unwired: 1 in]
      n345 = local read "light_21"() -> ()  [unwired: 1 in]
      n346 = local read "light_22"() -> ()  [unwired: 1 in]
      n347 = local read "light_23"() -> ()  [unwired: 1 in]
      n348 = local read "light_24"() -> ()  [unwired: 1 in]
      n349 = local read "light_25"() -> ()  [unwired: 1 in]
      n350 = local read "light_26"() -> ()  [unwired: 1 in]
      n351 = local read "light_27"() -> ()  [unwired: 1 in]
      n352 = local read "light_28"() -> ()  [unwired: 1 in]
      n353 = local read "light_29"() -> ()  [unwired: 1 in]
      n354 = local read "light_30"() -> ()  [unwired: 1 in]
      n355 = local read "light_31"() -> ()  [unwired: 1 in]
      n356 = local read "light_32"() -> ()  [unwired: 1 in]
      n357 = local read "light_33"() -> ()  [unwired: 1 in]
      n358 = local read "light_34"() -> ()  [unwired: 1 in]
      n359 = local read "light_35"() -> ()  [unwired: 1 in]
      n360 = local read "light_36"() -> ()  [unwired: 1 in]
      n361 = local read "light_37"() -> ()  [unwired: 1 in]
      n362 = local read "light_38"() -> ()  [unwired: 1 in]
      n363 = local read "light_39"() -> ()  [unwired: 1 in]
      n364 = local read "light_40"() -> ()  [unwired: 1 in]
      n365 = local read "light_41"() -> ()  [unwired: 1 in]
      n366 = local read "light_42"() -> ()  [unwired: 1 in]
      n367 = local read "light_43"() -> ()  [unwired: 1 in]
      n368 = local read "light_44"() -> ()  [unwired: 1 in]
      n369 = local read "light_45"() -> ()  [unwired: 1 in]
      n370 = local read "light_46"() -> ()  [unwired: 1 in]
      n371 = local read "light_47"() -> ()  [unwired: 1 in]
      n372 = local read "light_48"() -> ()  [unwired: 1 in]
      n373 = local read "light_49"() -> ()  [unwired: 1 in]
      n374 = local read "light_50"() -> ()  [unwired: 1 in]
      n375 = local read "light_51"() -> ()  [unwired: 1 in]
      n376 = local read "light_52"() -> ()  [unwired: 1 in]
      n377 = local read "light_53"() -> ()  [unwired: 1 in]
      n378 = local read "light_54"() -> ()  [unwired: 1 in]
      n379 = local read "light_55"() -> ()  [unwired: 1 in]
      n380 = local read "light_56"() -> ()  [unwired: 1 in]
      n381 = local read "light_57"() -> ()  [unwired: 1 in]
      n382 = local read "light_58"() -> ()  [unwired: 1 in]
      n383 = local read "light_59"() -> ()  [unwired: 1 in]
      n384 = local read "light_60"() -> ()  [unwired: 1 in]
      n385 = local read "light_61"() -> ()  [unwired: 1 in]
      n386 = local read "light_62"() -> ()  [unwired: 1 in]
      n387 = local read "light_63"() -> ()  [unwired: 1 in]
      n388 = local read "light_64"() -> ()  [unwired: 1 in]
      n389 = local read "light_65"() -> ()  [unwired: 1 in]
      n390 = local read "light_66"() -> ()  [unwired: 1 in]
      n391 = local read "light_67"() -> ()  [unwired: 1 in]
      n392 = local read "light_68"() -> ()  [unwired: 1 in]
      n393 = local read "light_69"() -> ()  [unwired: 1 in]
      n394 = local read "light_70"() -> ()  [unwired: 1 in]
      n395 = local read "light_71"() -> ()  [unwired: 1 in]
      n396 = local read "light_72"() -> ()  [unwired: 1 in]
      n397 = local read "light_73"() -> ()  [unwired: 1 in]
      n398 = local read "light_74"() -> ()  [unwired: 1 in]
      n399 = local read "light_75"() -> ()  [unwired: 1 in]
      n400 = local read "light_76"() -> ()  [unwired: 1 in]
      n401 = local read "light_77"() -> ()  [unwired: 1 in]
      n402 = local read "light_78"() -> ()  [unwired: 1 in]
      n403 = local read "light_79"() -> ()  [unwired: 1 in]
      n404 = local read "light_80"() -> ()  [unwired: 1 in]
    }
    frame Enabled {
    }
  }
  n405 = stacked-sequence {
    frame #0 {
      w31 = 0 ("同步_A1")
      w41 = T1."Disabled" ("禁用")
      n406 = property on="测试结论" class="Str"("Text.TextColor"=u32 0) -> ()  [unwired: 2 in, 2 out]
      n407 = local write "测试结论"("") -> ()
      n408 = local write "CAN端口"(u16 1 ("CAN端口")) -> ()
      n409 = local write "同步_A1"(w31) -> ()
      n410 = local write "同步_A2"(w31) -> ()
      n411 = property on="D_IN_1" class="Tbl (严格)"("DisabledEnum"=w41) -> ()  [unwired: 2 in, 2 out]
      n412 = property on="D_IN_2" class="Tbl (严格)"("DisabledEnum"=w41) -> ()  [unwired: 2 in, 2 out]
      n413 = property on="D_IN_3" class="Tbl (严格)"("DisabledEnum"=w41) -> ()  [unwired: 2 in, 2 out]
      n414 = property on="D_IN_4" class="Tbl (严格)"("DisabledEnum"=w41) -> ()  [unwired: 2 in, 2 out]
      n415 = property on="D_IN_5" class="Tbl (严格)"("DisabledEnum"=w41) -> ()  [unwired: 2 in, 2 out]
      n416 = property on="btn_开始试验" class="Bool"("DisabledEnum"=T1."Enabled" ("禁用")) -> ()  [unwired: 2 in, 2 out]
      n417 = Initialize Array("", 16 ("维数大小"), 4 ("维数大小")) -> (w37:string[][])
      n418 = local write "第几组数据"(0 ("第几组数据")) -> ()
      n419 = Initialize Array(enum16{"0", "1"}."0" ("输入值_32"), 80 ("维数大小")) -> (w28:enum16{"0", "1"}[])
      n420 = Initialize Array(FALSE, 80 ("维数大小")) -> (w24:bool[])
      n421 = Initialize Array(FALSE, 80 ("维数大小")) -> (w27:bool[])
      n422 = local write "关闭？"(FALSE) -> ()
      n423 = local write "数组_输入值"(w28) -> ()
      n424 = local write "数组_选择?"(w27) -> ()
      n425 = local write "D_IN_1"(w37) -> ()
      n426 = local write "D_IN_2"(w37) -> ()
      n427 = local write "D_IN_3"(w37) -> ()
      n428 = local write "D_IN_4"(w37) -> ()
      n429 = local write "D_IN_5"(w37) -> ()
      n430 = local write "合格？"(w24) -> ()
      n431 = for {
        N: 80 -> [_]
        tunnel: [w58] -> w22 mode=indexing
        tunnel: [w55] -> w21 mode=indexing
        tunnel: [w52] -> w20 mode=indexing
        tunnel: [w49] -> w19 mode=indexing
        tunnel: [w45] -> w18 mode=indexing
        i -> [w47]
        n432 = global read "试验配置信息.vi" "D_IN_3"() -> (w44:string[][])
        n433 = Index Array(array=w44, index (row)=w47, index (col)=1 ("禁用的索引 (列)")) -> (element=w57:string)
        n434 = Index Array(array=w44, index (row)=w47, index (col)=3 ("禁用的索引 (列)")) -> (element=w53:string)
        n435 = Index Array(array=w44, index (row)=w47, index (col)=5 ("禁用的索引 (列)")) -> (element=w46:string)
        n436 = Index Array(array=w44, index (row)=w47, index (col)=2 ("禁用的索引 (列)")) -> (element=w59:string)
        n437 = Index Array(array=w44, index (row)=w47, index (col)=4 ("禁用的索引 (列)")) -> (element=w50:string)
        n438 = Decimal String To Number(string=w57) -> (number=w55:i32)  [unwired: 2 in, 1 out]
        n439 = Decimal String To Number(string=w53) -> (number=w52:i32)  [unwired: 2 in, 1 out]
        n440 = Decimal String To Number(string=w46) -> (number=w45:i32)  [unwired: 2 in, 1 out]
        n441 = Decimal String To Number(string=w59) -> (number=w58:i32)  [unwired: 2 in, 1 out]
        n442 = Decimal String To Number(string=w50) -> (number=w49:i32)  [unwired: 2 in, 1 out]
      }
      n443 = global write "试验配置信息.vi" "设定输出通道"(w21) -> ()
      n444 = global write "试验配置信息.vi" "输出切换ID"(w20) -> ()
      n445 = global write "试验配置信息.vi" "跳变方向"(w18) -> ()
      n446 = global write "试验配置信息.vi" "设定输入通道"(w22) -> ()
      n447 = global write "试验配置信息.vi" "输入切换ID"(w19) -> ()
    }
  }
  n448 = Obtain Notifier(name (unnamed)=w6, notification data type=w6) -> (notifier out=w5:refnum<notifier>, error out=w1:errorcluster)  [unwired: 2 in, 1 out]
  n449 = while {
    tunnel: w5 -> [w62]
    tunnel: w1 -> [w61]
    stop <- w63 stop-if-true
    n450 = event shown="[13] \"btn_开始试验\": 值改变" {
      selector: _ -> [_ _ _ _ _ _ _ _ _ _ _ _ _ _ _ _ _ _]
      dyn-events: _ -> [_ _ _ _ _ _ _ _ _ _ _ _ _ _ _ _ _ _]
      timeout: _ -> [_ _ _ _ _ _ _ _ _ _ _ _ _ _ _ _ _ _]
      tunnel: [_ w64 w65 _ _ _ _ _ _ _ _ _ _ _ _ _ _ _] -> w63
      tunnel: w62 -> [_ _ _ _ _ _ _ _ _ _ _ _ _ w107 _ _ _ _]
      tunnel: w61 -> [_ _ _ _ _ _ _ _ _ _ _ _ _ w106 _ _ _ _]
      event Timeout {
        n451 = event-data() -> ()  [unwired: 1 in, 2 out]
      }
      event Panel Close {
        w64 = TRUE ("关闭？")
        n452 = event-data() -> ()  [unwired: 1 in, 3 out]
        n453 = local write "关闭？"(w64) -> ()
      }
      event "btn_关闭": Value Change {
        w65 = TRUE
        n454 = event-data() -> ()  [unwired: 1 in, 5 out]
        n455 = local write "关闭？"(w65) -> ()
      }
      event "btn_全选_1": Value Change {
        n456 = event-data() -> ("NewVal"=w67:bool)  [unwired: 1 in, 4 out]
        n457 = case shown="假" w67 {
          tunnel: [FALSE ("单选_第41路") TRUE ("单选_第41路")] -> w66
          frame False {
          }
          frame True {
          }
        }
        n458 = local write "单选_第1路"(w66) -> ()
        n459 = local write "单选_第2路"(w66) -> ()
        n460 = local write "单选_第3路"(w66) -> ()
        n461 = local write "单选_第4路"(w66) -> ()
        n462 = local write "单选_第5路"(w66) -> ()
        n463 = local write "单选_第6路"(w66) -> ()
        n464 = local write "单选_第7路"(w66) -> ()
        n465 = local write "单选_第8路"(w66) -> ()
        n466 = local write "单选_第9路"(w66) -> ()
        n467 = local write "单选_第10路"(w66) -> ()
        n468 = local write "单选_第11路"(w66) -> ()
        n469 = local write "单选_第12路"(w66) -> ()
        n470 = local write "单选_第13路"(w66) -> ()
        n471 = local write "单选_第14路"(w66) -> ()
        n472 = local write "单选_第15路"(w66) -> ()
        n473 = local write "单选_第16路"(w66) -> ()
      }
      event "btn_全选_2": Value Change {
        n474 = event-data() -> ("NewVal"=w71:bool)  [unwired: 1 in, 4 out]
        n475 = case shown="假" w71 {
          tunnel: [FALSE ("单选_第41路") TRUE ("单选_第41路")] -> w70
          frame False {
          }
          frame True {
          }
        }
        n476 = local write "单选_第17路"(w70) -> ()
        n477 = local write "单选_第18路"(w70) -> ()
        n478 = local write "单选_第19路"(w70) -> ()
        n479 = local write "单选_第20路"(w70) -> ()
        n480 = local write "单选_第21路"(w70) -> ()
        n481 = local write "单选_第22路"(w70) -> ()
        n482 = local write "单选_第23路"(w70) -> ()
        n483 = local write "单选_第24路"(w70) -> ()
        n484 = local write "单选_第25路"(w70) -> ()
        n485 = local write "单选_第26路"(w70) -> ()
        n486 = local write "单选_第27路"(w70) -> ()
        n487 = local write "单选_第28路"(w70) -> ()
        n488 = local write "单选_第29路"(w70) -> ()
        n489 = local write "单选_第30路"(w70) -> ()
        n490 = local write "单选_第31路"(w70) -> ()
        n491 = local write "单选_第32路"(w70) -> ()
      }
      event "btn_全选_3": Value Change {
        n492 = event-data() -> ("NewVal"=w75:bool)  [unwired: 1 in, 4 out]
        n493 = case shown="假" w75 {
          tunnel: [FALSE ("单选_第41路") TRUE ("单选_第41路")] -> w74
          frame False {
          }
          frame True {
          }
        }
        n494 = local write "单选_第33路"(w74) -> ()
        n495 = local write "单选_第34路"(w74) -> ()
        n496 = local write "单选_第35路"(w74) -> ()
        n497 = local write "单选_第36路"(w74) -> ()
        n498 = local write "单选_第37路"(w74) -> ()
        n499 = local write "单选_第38路"(w74) -> ()
        n500 = local write "单选_第39路"(w74) -> ()
        n501 = local write "单选_第40路"(w74) -> ()
        n502 = local write "单选_第41路"(w74) -> ()
        n503 = local write "单选_第42路"(w74) -> ()
        n504 = local write "单选_第43路"(w74) -> ()
        n505 = local write "单选_第44路"(w74) -> ()
        n506 = local write "单选_第45路"(w74) -> ()
        n507 = local write "单选_第46路"(w74) -> ()
        n508 = local write "单选_第47路"(w74) -> ()
        n509 = local write "单选_第48路"(w74) -> ()
      }
      event "btn_全选_4": Value Change {
        n510 = event-data() -> ("NewVal"=w79:bool)  [unwired: 1 in, 4 out]
        n511 = case shown="假" w79 {
          tunnel: [FALSE ("单选_第41路") TRUE ("单选_第41路")] -> w78
          frame False {
          }
          frame True {
          }
        }
        n512 = local write "单选_第49路"(w78) -> ()
        n513 = local write "单选_第50路"(w78) -> ()
        n514 = local write "单选_第51路"(w78) -> ()
        n515 = local write "单选_第52路"(w78) -> ()
        n516 = local write "单选_第53路"(w78) -> ()
        n517 = local write "单选_第54路"(w78) -> ()
        n518 = local write "单选_第55路"(w78) -> ()
        n519 = local write "单选_第56路"(w78) -> ()
        n520 = local write "单选_第57路"(w78) -> ()
        n521 = local write "单选_第58路"(w78) -> ()
        n522 = local write "单选_第59路"(w78) -> ()
        n523 = local write "单选_第60路"(w78) -> ()
        n524 = local write "单选_第61路"(w78) -> ()
        n525 = local write "单选_第62路"(w78) -> ()
        n526 = local write "单选_第63路"(w78) -> ()
        n527 = local write "单选_第64路"(w78) -> ()
      }
      event "btn_全选_5": Value Change {
        n528 = event-data() -> ("NewVal"=w83:bool)  [unwired: 1 in, 4 out]
        n529 = case shown="假" w83 {
          tunnel: [FALSE ("单选_第41路") TRUE ("单选_第41路")] -> w82
          frame False {
          }
          frame True {
          }
        }
        n530 = local write "单选_第71路"(w82) -> ()
        n531 = local write "单选_第79路"(w82) -> ()
        n532 = local write "单选_第65路"(w82) -> ()
        n533 = local write "单选_第66路"(w82) -> ()
        n534 = local write "单选_第67路"(w82) -> ()
        n535 = local write "单选_第68路"(w82) -> ()
        n536 = local write "单选_第69路"(w82) -> ()
        n537 = local write "单选_第70路"(w82) -> ()
        n538 = local write "单选_第72路"(w82) -> ()
        n539 = local write "单选_第73路"(w82) -> ()
        n540 = local write "单选_第74路"(w82) -> ()
        n541 = local write "单选_第75路"(w82) -> ()
        n542 = local write "单选_第76路"(w82) -> ()
        n543 = local write "单选_第77路"(w82) -> ()
        n544 = local write "单选_第78路"(w82) -> ()
        n545 = local write "单选_第80路"(w82) -> ()
      }
      event "btn_置1_1": Value Change {
        n546 = event-data() -> ("NewVal"=w87:bool)  [unwired: 1 in, 4 out]
        n547 = case shown="假" w87 {
          tunnel: [enum16{"0", "1"}."0" ("输入值_41") enum16{"0", "1"}."1" ("输入值_41")] -> w86
          frame False {
          }
          frame True {
          }
        }
        n548 = local write "输入值_1"(w86) -> ()
        n549 = local write "输入值_2"(w86) -> ()
        n550 = local write "输入值_3"(w86) -> ()
        n551 = local write "输入值_4"(w86) -> ()
        n552 = local write "输入值_5"(w86) -> ()
        n553 = local write "输入值_6"(w86) -> ()
        n554 = local write "输入值_7"(w86) -> ()
        n555 = local write "输入值_8"(w86) -> ()
        n556 = local write "输入值_9"(w86) -> ()
        n557 = local write "输入值_10"(w86) -> ()
        n558 = local write "输入值_11"(w86) -> ()
        n559 = local write "输入值_12"(w86) -> ()
        n560 = local write "输入值_13"(w86) -> ()
        n561 = local write "输入值_14"(w86) -> ()
        n562 = local write "输入值_15"(w86) -> ()
        n563 = local write "输入值_16"(w86) -> ()
      }
      event "btn_置1_2": Value Change {
        n564 = event-data() -> ("NewVal"=w91:bool)  [unwired: 1 in, 4 out]
        n565 = case shown="假" w91 {
          tunnel: [enum16{"0", "1"}."0" ("输入值_41") enum16{"0", "1"}."1" ("输入值_41")] -> w90
          frame False {
          }
          frame True {
          }
        }
        n566 = local write "输入值_17"(w90) -> ()
        n567 = local write "输入值_18"(w90) -> ()
        n568 = local write "输入值_19"(w90) -> ()
        n569 = local write "输入值_20"(w90) -> ()
        n570 = local write "输入值_21"(w90) -> ()
        n571 = local write "输入值_22"(w90) -> ()
        n572 = local write "输入值_23"(w90) -> ()
        n573 = local write "输入值_24"(w90) -> ()
        n574 = local write "输入值_25"(w90) -> ()
        n575 = local write "输入值_26"(w90) -> ()
        n576 = local write "输入值_27"(w90) -> ()
        n577 = local write "输入值_28"(w90) -> ()
        n578 = local write "输入值_29"(w90) -> ()
        n579 = local write "输入值_30"(w90) -> ()
        n580 = local write "输入值_31"(w90) -> ()
        n581 = local write "输入值_32"(w90) -> ()
      }
      event "btn_置1_3": Value Change {
        n582 = event-data() -> ("NewVal"=w95:bool)  [unwired: 1 in, 4 out]
        n583 = case shown="假" w95 {
          tunnel: [enum16{"0", "1"}."0" ("输入值_41") enum16{"0", "1"}."1" ("输入值_41")] -> w94
          frame False {
          }
          frame True {
          }
        }
        n584 = local write "输入值_33"(w94) -> ()
        n585 = local write "输入值_34"(w94) -> ()
        n586 = local write "输入值_35"(w94) -> ()
        n587 = local write "输入值_36"(w94) -> ()
        n588 = local write "输入值_37"(w94) -> ()
        n589 = local write "输入值_38"(w94) -> ()
        n590 = local write "输入值_39"(w94) -> ()
        n591 = local write "输入值_40"(w94) -> ()
        n592 = local write "输入值_41"(w94) -> ()
        n593 = local write "输入值_42"(w94) -> ()
        n594 = local write "输入值_43"(w94) -> ()
        n595 = local write "输入值_44"(w94) -> ()
        n596 = local write "输入值_45"(w94) -> ()
        n597 = local write "输入值_46"(w94) -> ()
        n598 = local write "输入值_47"(w94) -> ()
        n599 = local write "输入值_48"(w94) -> ()
      }
      event "btn_置1_4": Value Change {
        n600 = event-data() -> ("NewVal"=w99:bool)  [unwired: 1 in, 4 out]
        n601 = case shown="假" w99 {
          tunnel: [enum16{"0", "1"}."0" ("输入值_41") enum16{"0", "1"}."1" ("输入值_41")] -> w98
          frame False {
          }
          frame True {
          }
        }
        n602 = local write "输入值_49"(w98) -> ()
        n603 = local write "输入值_50"(w98) -> ()
        n604 = local write "输入值_51"(w98) -> ()
        n605 = local write "输入值_52"(w98) -> ()
        n606 = local write "输入值_53"(w98) -> ()
        n607 = local write "输入值_54"(w98) -> ()
        n608 = local write "输入值_55"(w98) -> ()
        n609 = local write "输入值_56"(w98) -> ()
        n610 = local write "输入值_57"(w98) -> ()
        n611 = local write "输入值_58"(w98) -> ()
        n612 = local write "输入值_59"(w98) -> ()
        n613 = local write "输入值_60"(w98) -> ()
        n614 = local write "输入值_61"(w98) -> ()
        n615 = local write "输入值_62"(w98) -> ()
        n616 = local write "输入值_63"(w98) -> ()
        n617 = local write "输入值_64"(w98) -> ()
      }
      event "btn_置1_5": Value Change {
        n618 = event-data() -> ("NewVal"=w103:bool)  [unwired: 1 in, 4 out]
        n619 = case shown="假" w103 {
          tunnel: [enum16{"0", "1"}."0" ("输入值_41") enum16{"0", "1"}."1" ("输入值_41")] -> w102
          frame False {
          }
          frame True {
          }
        }
        n620 = local write "输入值_65"(w102) -> ()
        n621 = local write "输入值_66"(w102) -> ()
        n622 = local write "输入值_67"(w102) -> ()
        n623 = local write "输入值_68"(w102) -> ()
        n624 = local write "输入值_69"(w102) -> ()
        n625 = local write "输入值_70"(w102) -> ()
        n626 = local write "输入值_71"(w102) -> ()
        n627 = local write "输入值_72"(w102) -> ()
        n628 = local write "输入值_73"(w102) -> ()
        n629 = local write "输入值_74"(w102) -> ()
        n630 = local write "输入值_75"(w102) -> ()
        n631 = local write "输入值_76"(w102) -> ()
        n632 = local write "输入值_77"(w102) -> ()
        n633 = local write "输入值_78"(w102) -> ()
        n634 = local write "输入值_79"(w102) -> ()
        n635 = local write "输入值_80"(w102) -> ()
      }
      event "btn_开始试验": Value Change {
        n636 = event-data() -> ()  [unwired: 1 in, 5 out]
        n637 = stacked-sequence {
          tunnel: w107 -> [_ _ w303]
          tunnel: w106 -> [_ _ w302]
          frame #0 {
            w122 = 0 ("同步_A1")
            n638 = stacked-sequence {
              tunnel: [w127 _ _ _ _] -> w119
              tunnel: [w126 _ _ _ _] -> w113
              tunnel: [_ w161 _ _ _] -> w118
              tunnel: [_ w160 _ _ _] -> w112
              tunnel: [_ _ w195 _ _] -> w117
              tunnel: [_ _ w194 _ _] -> w111
              tunnel: [_ _ _ w229 _] -> w116
              tunnel: [_ _ _ w228 _] -> w110
              tunnel: [_ _ _ _ w263] -> w115
              tunnel: [_ _ _ _ w262] -> w109
              frame #0 {
                n639 = local read "单选_第1路"() -> (w144:bool)
                n640 = local read "单选_第2路"() -> (w145:bool)
                n641 = local read "单选_第3路"() -> (w146:bool)
                n642 = local read "单选_第4路"() -> (w147:bool)
                n643 = local read "单选_第5路"() -> (w148:bool)
                n644 = local read "单选_第6路"() -> (w149:bool)
                n645 = local read "单选_第7路"() -> (w150:bool)
                n646 = local read "单选_第8路"() -> (w151:bool)
                n647 = local read "单选_第9路"() -> (w152:bool)
                n648 = local read "单选_第10路"() -> (w153:bool)
                n649 = local read "单选_第11路"() -> (w154:bool)
                n650 = local read "单选_第12路"() -> (w155:bool)
                n651 = local read "单选_第13路"() -> (w156:bool)
                n652 = local read "单选_第14路"() -> (w157:bool)
                n653 = local read "单选_第15路"() -> (w158:bool)
                n654 = local read "单选_第16路"() -> (w159:bool)
                n655 = local read "输入值_1"() -> (w128:enum16{"0", "1"})
                n656 = local read "输入值_2"() -> (w129:enum16{"0", "1"})
                n657 = local read "输入值_3"() -> (w130:enum16{"0", "1"})
                n658 = local read "输入值_4"() -> (w131:enum16{"0", "1"})
                n659 = local read "输入值_5"() -> (w132:enum16{"0", "1"})
                n660 = local read "输入值_6"() -> (w133:enum16{"0", "1"})
                n661 = local read "输入值_7"() -> (w134:enum16{"0", "1"})
                n662 = local read "输入值_8"() -> (w135:enum16{"0", "1"})
                n663 = local read "输入值_9"() -> (w136:enum16{"0", "1"})
                n664 = local read "输入值_10"() -> (w137:enum16{"0", "1"})
                n665 = local read "输入值_11"() -> (w138:enum16{"0", "1"})
                n666 = local read "输入值_12"() -> (w139:enum16{"0", "1"})
                n667 = local read "输入值_13"() -> (w140:enum16{"0", "1"})
                n668 = local read "输入值_14"() -> (w141:enum16{"0", "1"})
                n669 = local read "输入值_15"() -> (w142:enum16{"0", "1"})
                n670 = local read "输入值_16"() -> (w143:enum16{"0", "1"})
                n671 = Build Array(w144, w145, w146, w147, w148, w149, w150, w151, w152, w153, w154, w155, w156, w157, w158, w159) -> (w127:bool[])
                n672 = Build Array(w128, w129, w130, w131, w132, w133, w134, w135, w136, w137, w138, w139, w140, w141, w142, w143) -> (w126:enum16{"0", "1"}[])
              }
              frame #1 {
                n673 = local read "单选_第17路"() -> (w178:bool)
                n674 = local read "单选_第18路"() -> (w179:bool)
                n675 = local read "单选_第19路"() -> (w180:bool)
                n676 = local read "单选_第20路"() -> (w181:bool)
                n677 = local read "单选_第21路"() -> (w182:bool)
                n678 = local read "单选_第22路"() -> (w183:bool)
                n679 = local read "单选_第23路"() -> (w184:bool)
                n680 = local read "单选_第24路"() -> (w185:bool)
                n681 = local read "单选_第25路"() -> (w186:bool)
                n682 = local read "单选_第26路"() -> (w187:bool)
                n683 = local read "单选_第27路"() -> (w188:bool)
                n684 = local read "单选_第28路"() -> (w189:bool)
                n685 = local read "单选_第29路"() -> (w190:bool)
                n686 = local read "单选_第30路"() -> (w191:bool)
                n687 = local read "单选_第31路"() -> (w192:bool)
                n688 = local read "单选_第32路"() -> (w193:bool)
                n689 = local read "输入值_17"() -> (w162:enum16{"0", "1"})
                n690 = local read "输入值_18"() -> (w163:enum16{"0", "1"})
                n691 = local read "输入值_19"() -> (w164:enum16{"0", "1"})
                n692 = local read "输入值_20"() -> (w165:enum16{"0", "1"})
                n693 = local read "输入值_21"() -> (w166:enum16{"0", "1"})
                n694 = local read "输入值_22"() -> (w167:enum16{"0", "1"})
                n695 = local read "输入值_23"() -> (w168:enum16{"0", "1"})
                n696 = local read "输入值_24"() -> (w169:enum16{"0", "1"})
                n697 = local read "输入值_25"() -> (w170:enum16{"0", "1"})
                n698 = local read "输入值_26"() -> (w171:enum16{"0", "1"})
                n699 = local read "输入值_27"() -> (w172:enum16{"0", "1"})
                n700 = local read "输入值_28"() -> (w173:enum16{"0", "1"})
                n701 = local read "输入值_29"() -> (w174:enum16{"0", "1"})
                n702 = local read "输入值_30"() -> (w175:enum16{"0", "1"})
                n703 = local read "输入值_31"() -> (w176:enum16{"0", "1"})
                n704 = local read "输入值_32"() -> (w177:enum16{"0", "1"})
                n705 = Build Array(w178, w179, w180, w181, w182, w183, w184, w185, w186, w187, w188, w189, w190, w191, w192, w193) -> (w161:bool[])
                n706 = Build Array(w162, w163, w164, w165, w166, w167, w168, w169, w170, w171, w172, w173, w174, w175, w176, w177) -> (w160:enum16{"0", "1"}[])
              }
              frame #2 {
                n707 = local read "单选_第33路"() -> (w212:bool)
                n708 = local read "单选_第34路"() -> (w213:bool)
                n709 = local read "单选_第35路"() -> (w214:bool)
                n710 = local read "单选_第36路"() -> (w215:bool)
                n711 = local read "单选_第37路"() -> (w216:bool)
                n712 = local read "单选_第38路"() -> (w217:bool)
                n713 = local read "单选_第39路"() -> (w218:bool)
                n714 = local read "单选_第40路"() -> (w219:bool)
                n715 = local read "单选_第41路"() -> (w220:bool)
                n716 = local read "单选_第42路"() -> (w221:bool)
                n717 = local read "单选_第43路"() -> (w222:bool)
                n718 = local read "单选_第44路"() -> (w223:bool)
                n719 = local read "单选_第45路"() -> (w224:bool)
                n720 = local read "单选_第46路"() -> (w225:bool)
                n721 = local read "单选_第47路"() -> (w226:bool)
                n722 = local read "单选_第48路"() -> (w227:bool)
                n723 = local read "输入值_33"() -> (w196:enum16{"0", "1"})
                n724 = local read "输入值_34"() -> (w197:enum16{"0", "1"})
                n725 = local read "输入值_35"() -> (w198:enum16{"0", "1"})
                n726 = local read "输入值_36"() -> (w199:enum16{"0", "1"})
                n727 = local read "输入值_37"() -> (w200:enum16{"0", "1"})
                n728 = local read "输入值_38"() -> (w201:enum16{"0", "1"})
                n729 = local read "输入值_39"() -> (w202:enum16{"0", "1"})
                n730 = local read "输入值_40"() -> (w203:enum16{"0", "1"})
                n731 = local read "输入值_41"() -> (w204:enum16{"0", "1"})
                n732 = local read "输入值_42"() -> (w205:enum16{"0", "1"})
                n733 = local read "输入值_43"() -> (w206:enum16{"0", "1"})
                n734 = local read "输入值_44"() -> (w207:enum16{"0", "1"})
                n735 = local read "输入值_45"() -> (w208:enum16{"0", "1"})
                n736 = local read "输入值_46"() -> (w209:enum16{"0", "1"})
                n737 = local read "输入值_47"() -> (w210:enum16{"0", "1"})
                n738 = local read "输入值_48"() -> (w211:enum16{"0", "1"})
                n739 = Build Array(w196, w197, w198, w199, w200, w201, w202, w203, w204, w205, w206, w207, w208, w209, w210, w211) -> (w194:enum16{"0", "1"}[])
                n740 = Build Array(w212, w213, w214, w215, w216, w217, w218, w219, w220, w221, w222, w223, w224, w225, w226, w227) -> (w195:bool[])
              }
              frame #3 {
                n741 = local read "单选_第49路"() -> (w246:bool)
                n742 = local read "单选_第50路"() -> (w247:bool)
                n743 = local read "单选_第51路"() -> (w248:bool)
                n744 = local read "单选_第52路"() -> (w249:bool)
                n745 = local read "单选_第53路"() -> (w250:bool)
                n746 = local read "单选_第54路"() -> (w251:bool)
                n747 = local read "单选_第55路"() -> (w252:bool)
                n748 = local read "单选_第56路"() -> (w253:bool)
                n749 = local read "单选_第57路"() -> (w254:bool)
                n750 = local read "单选_第58路"() -> (w255:bool)
                n751 = local read "单选_第59路"() -> (w256:bool)
                n752 = local read "单选_第60路"() -> (w257:bool)
                n753 = local read "单选_第61路"() -> (w258:bool)
                n754 = local read "单选_第62路"() -> (w259:bool)
                n755 = local read "单选_第63路"() -> (w260:bool)
                n756 = local read "单选_第64路"() -> (w261:bool)
                n757 = local read "输入值_49"() -> (w230:enum16{"0", "1"})
                n758 = local read "输入值_50"() -> (w231:enum16{"0", "1"})
                n759 = local read "输入值_51"() -> (w232:enum16{"0", "1"})
                n760 = local read "输入值_52"() -> (w233:enum16{"0", "1"})
                n761 = local read "输入值_53"() -> (w234:enum16{"0", "1"})
                n762 = local read "输入值_54"() -> (w235:enum16{"0", "1"})
                n763 = local read "输入值_55"() -> (w236:enum16{"0", "1"})
                n764 = local read "输入值_56"() -> (w237:enum16{"0", "1"})
                n765 = local read "输入值_57"() -> (w238:enum16{"0", "1"})
                n766 = local read "输入值_58"() -> (w239:enum16{"0", "1"})
                n767 = local read "输入值_59"() -> (w240:enum16{"0", "1"})
                n768 = local read "输入值_60"() -> (w241:enum16{"0", "1"})
                n769 = local read "输入值_61"() -> (w242:enum16{"0", "1"})
                n770 = local read "输入值_62"() -> (w243:enum16{"0", "1"})
                n771 = local read "输入值_63"() -> (w244:enum16{"0", "1"})
                n772 = local read "输入值_64"() -> (w245:enum16{"0", "1"})
                n773 = Build Array(w246, w247, w248, w249, w250, w251, w252, w253, w254, w255, w256, w257, w258, w259, w260, w261) -> (w229:bool[])
                n774 = Build Array(w230, w231, w232, w233, w234, w235, w236, w237, w238, w239, w240, w241, w242, w243, w244, w245) -> (w228:enum16{"0", "1"}[])
              }
              frame #4 {
                n775 = local read "单选_第71路"() -> (w286:bool)
                n776 = local read "单选_第79路"() -> (w294:bool)
                n777 = local read "单选_第65路"() -> (w280:bool)
                n778 = local read "单选_第66路"() -> (w281:bool)
                n779 = local read "单选_第67路"() -> (w282:bool)
                n780 = local read "单选_第68路"() -> (w283:bool)
                n781 = local read "单选_第69路"() -> (w284:bool)
                n782 = local read "单选_第70路"() -> (w285:bool)
                n783 = local read "单选_第72路"() -> (w287:bool)
                n784 = local read "单选_第73路"() -> (w288:bool)
                n785 = local read "单选_第74路"() -> (w289:bool)
                n786 = local read "单选_第75路"() -> (w290:bool)
                n787 = local read "单选_第76路"() -> (w291:bool)
                n788 = local read "单选_第77路"() -> (w292:bool)
                n789 = local read "单选_第78路"() -> (w293:bool)
                n790 = local read "单选_第80路"() -> (w295:bool)
                n791 = local read "输入值_65"() -> (w264:enum16{"0", "1"})
                n792 = local read "输入值_66"() -> (w265:enum16{"0", "1"})
                n793 = local read "输入值_67"() -> (w266:enum16{"0", "1"})
                n794 = local read "输入值_68"() -> (w267:enum16{"0", "1"})
                n795 = local read "输入值_69"() -> (w268:enum16{"0", "1"})
                n796 = local read "输入值_70"() -> (w269:enum16{"0", "1"})
                n797 = local read "输入值_71"() -> (w270:enum16{"0", "1"})
                n798 = local read "输入值_72"() -> (w271:enum16{"0", "1"})
                n799 = local read "输入值_73"() -> (w272:enum16{"0", "1"})
                n800 = local read "输入值_74"() -> (w273:enum16{"0", "1"})
                n801 = local read "输入值_75"() -> (w274:enum16{"0", "1"})
                n802 = local read "输入值_76"() -> (w275:enum16{"0", "1"})
                n803 = local read "输入值_77"() -> (w276:enum16{"0", "1"})
                n804 = local read "输入值_78"() -> (w277:enum16{"0", "1"})
                n805 = local read "输入值_79"() -> (w278:enum16{"0", "1"})
                n806 = local read "输入值_80"() -> (w279:enum16{"0", "1"})
                n807 = Build Array(w264, w265, w266, w267, w268, w269, w270, w271, w272, w273, w274, w275, w276, w277, w278, w279) -> (w262:enum16{"0", "1"}[])
                n808 = Build Array(w280, w281, w282, w283, w284, w285, w286, w287, w288, w289, w290, w291, w292, w293, w294, w295) -> (w263:bool[])
              }
            }
            n809 = local read "数组_输入值"() -> (w124:enum16{"0", "1"}[])
            n810 = local read "数组_选择?"() -> (w125:bool[])
            n811 = local write "测试结论"("") -> ()
            n812 = local write "同步_A1"(w122) -> ()
            n813 = local write "同步_A2"(w122) -> ()
            n814 = Insert Into Array(array=w124, index=0 ("索引 (行)"), new element #1=w113, new element #2=w112, new element #3=w111, new element #4=w110, new element #5=w109) -> (w123:enum16{"0", "1"}[])
            n815 = Insert Into Array(array=w125, index=0 ("索引 (行)"), new element #1=w119, new element #2=w118, new element #3=w117, new element #4=w116, new element #5=w115) -> (w108:bool[])
            n816 = local write "数组_输入值"(w123) -> ()
            n817 = local write "数组_选择?"(w108) -> ()
            n818 = Or Array Elements(Boolean array=w108) -> ()  [unwired: 1 out]
          }
          frame #1 {
            w297 = cluster{u32, u32}[] [{9868950, 9868950}]
            n819 = property on="light_1" class="Bool (严格)"("Colors [4]"=w297) -> ()  [unwired: 2 in, 2 out]
            n820 = property on="light_2" class="Bool (严格)"("Colors [4]"=w297) -> ()  [unwired: 2 in, 2 out]
            n821 = property on="light_3" class="Bool (严格)"("Colors [4]"=w297) -> ()  [unwired: 2 in, 2 out]
            n822 = property on="light_4" class="Bool (严格)"("Colors [4]"=w297) -> ()  [unwired: 2 in, 2 out]
            n823 = property on="light_5" class="Bool (严格)"("Colors [4]"=w297) -> ()  [unwired: 2 in, 2 out]
            n824 = property on="light_6" class="Bool (严格)"("Colors [4]"=w297) -> ()  [unwired: 2 in, 2 out]
            n825 = property on="light_7" class="Bool (严格)"("Colors [4]"=w297) -> ()  [unwired: 2 in, 2 out]
            n826 = property on="light_8" class="Bool (严格)"("Colors [4]"=w297) -> ()  [unwired: 2 in, 2 out]
            n827 = property on="light_9" class="Bool (严格)"("Colors [4]"=w297) -> ()  [unwired: 2 in, 2 out]
            n828 = property on="light_10" class="Bool (严格)"("Colors [4]"=w297) -> ()  [unwired: 2 in, 2 out]
            n829 = property on="light_11" class="Bool (严格)"("Colors [4]"=w297) -> ()  [unwired: 2 in, 2 out]
            n830 = property on="light_12" class="Bool (严格)"("Colors [4]"=w297) -> ()  [unwired: 2 in, 2 out]
            n831 = property on="light_13" class="Bool (严格)"("Colors [4]"=w297) -> ()  [unwired: 2 in, 2 out]
            n832 = property on="light_14" class="Bool (严格)"("Colors [4]"=w297) -> ()  [unwired: 2 in, 2 out]
            n833 = property on="light_15" class="Bool (严格)"("Colors [4]"=w297) -> ()  [unwired: 2 in, 2 out]
            n834 = property on="light_16" class="Bool (严格)"("Colors [4]"=w297) -> ()  [unwired: 2 in, 2 out]
            n835 = property on="light_17" class="Bool (严格)"("Colors [4]"=w297) -> ()  [unwired: 2 in, 2 out]
            n836 = property on="light_18" class="Bool (严格)"("Colors [4]"=w297) -> ()  [unwired: 2 in, 2 out]
            n837 = property on="light_19" class="Bool (严格)"("Colors [4]"=w297) -> ()  [unwired: 2 in, 2 out]
            n838 = property on="light_20" class="Bool (严格)"("Colors [4]"=w297) -> ()  [unwired: 2 in, 2 out]
            n839 = property on="light_21" class="Bool (严格)"("Colors [4]"=w297) -> ()  [unwired: 2 in, 2 out]
            n840 = property on="light_22" class="Bool (严格)"("Colors [4]"=w297) -> ()  [unwired: 2 in, 2 out]
            n841 = property on="light_23" class="Bool (严格)"("Colors [4]"=w297) -> ()  [unwired: 2 in, 2 out]
            n842 = property on="light_24" class="Bool (严格)"("Colors [4]"=w297) -> ()  [unwired: 2 in, 2 out]
            n843 = property on="light_25" class="Bool (严格)"("Colors [4]"=w297) -> ()  [unwired: 2 in, 2 out]
            n844 = property on="light_26" class="Bool (严格)"("Colors [4]"=w297) -> ()  [unwired: 2 in, 2 out]
            n845 = property on="light_27" class="Bool (严格)"("Colors [4]"=w297) -> ()  [unwired: 2 in, 2 out]
            n846 = property on="light_28" class="Bool (严格)"("Colors [4]"=w297) -> ()  [unwired: 2 in, 2 out]
            n847 = property on="light_29" class="Bool (严格)"("Colors [4]"=w297) -> ()  [unwired: 2 in, 2 out]
            n848 = property on="light_30" class="Bool (严格)"("Colors [4]"=w297) -> ()  [unwired: 2 in, 2 out]
            n849 = property on="light_31" class="Bool (严格)"("Colors [4]"=w297) -> ()  [unwired: 2 in, 2 out]
            n850 = property on="light_32" class="Bool (严格)"("Colors [4]"=w297) -> ()  [unwired: 2 in, 2 out]
            n851 = property on="light_33" class="Bool (严格)"("Colors [4]"=w297) -> ()  [unwired: 2 in, 2 out]
            n852 = property on="light_34" class="Bool (严格)"("Colors [4]"=w297) -> ()  [unwired: 2 in, 2 out]
            n853 = property on="light_35" class="Bool (严格)"("Colors [4]"=w297) -> ()  [unwired: 2 in, 2 out]
            n854 = property on="light_36" class="Bool (严格)"("Colors [4]"=w297) -> ()  [unwired: 2 in, 2 out]
            n855 = property on="light_37" class="Bool (严格)"("Colors [4]"=w297) -> ()  [unwired: 2 in, 2 out]
            n856 = property on="light_38" class="Bool (严格)"("Colors [4]"=w297) -> ()  [unwired: 2 in, 2 out]
            n857 = property on="light_39" class="Bool (严格)"("Colors [4]"=w297) -> ()  [unwired: 2 in, 2 out]
            n858 = property on="light_40" class="Bool (严格)"("Colors [4]"=w297) -> ()  [unwired: 2 in, 2 out]
            n859 = property on="light_41" class="Bool (严格)"("Colors [4]"=w297) -> ()  [unwired: 2 in, 2 out]
            n860 = property on="light_42" class="Bool (严格)"("Colors [4]"=w297) -> ()  [unwired: 2 in, 2 out]
            n861 = property on="light_43" class="Bool (严格)"("Colors [4]"=w297) -> ()  [unwired: 2 in, 2 out]
            n862 = property on="light_44" class="Bool (严格)"("Colors [4]"=w297) -> ()  [unwired: 2 in, 2 out]
            n863 = property on="light_45" class="Bool (严格)"("Colors [4]"=w297) -> ()  [unwired: 2 in, 2 out]
            n864 = property on="light_46" class="Bool (严格)"("Colors [4]"=w297) -> ()  [unwired: 2 in, 2 out]
            n865 = property on="light_47" class="Bool (严格)"("Colors [4]"=w297) -> ()  [unwired: 2 in, 2 out]
            n866 = property on="light_48" class="Bool (严格)"("Colors [4]"=w297) -> ()  [unwired: 2 in, 2 out]
            n867 = property on="light_49" class="Bool (严格)"("Colors [4]"=w297) -> ()  [unwired: 2 in, 2 out]
            n868 = property on="light_50" class="Bool (严格)"("Colors [4]"=w297) -> ()  [unwired: 2 in, 2 out]
            n869 = property on="light_51" class="Bool (严格)"("Colors [4]"=w297) -> ()  [unwired: 2 in, 2 out]
            n870 = property on="light_52" class="Bool (严格)"("Colors [4]"=w297) -> ()  [unwired: 2 in, 2 out]
            n871 = property on="light_53" class="Bool (严格)"("Colors [4]"=w297) -> ()  [unwired: 2 in, 2 out]
            n872 = property on="light_54" class="Bool (严格)"("Colors [4]"=w297) -> ()  [unwired: 2 in, 2 out]
            n873 = property on="light_55" class="Bool (严格)"("Colors [4]"=w297) -> ()  [unwired: 2 in, 2 out]
            n874 = property on="light_56" class="Bool (严格)"("Colors [4]"=w297) -> ()  [unwired: 2 in, 2 out]
            n875 = property on="light_57" class="Bool (严格)"("Colors [4]"=w297) -> ()  [unwired: 2 in, 2 out]
            n876 = property on="light_58" class="Bool (严格)"("Colors [4]"=w297) -> ()  [unwired: 2 in, 2 out]
            n877 = property on="light_59" class="Bool (严格)"("Colors [4]"=w297) -> ()  [unwired: 2 in, 2 out]
            n878 = property on="light_60" class="Bool (严格)"("Colors [4]"=w297) -> ()  [unwired: 2 in, 2 out]
            n879 = property on="light_61" class="Bool (严格)"("Colors [4]"=w297) -> ()  [unwired: 2 in, 2 out]
            n880 = property on="light_62" class="Bool (严格)"("Colors [4]"=w297) -> ()  [unwired: 2 in, 2 out]
            n881 = property on="light_63" class="Bool (严格)"("Colors [4]"=w297) -> ()  [unwired: 2 in, 2 out]
            n882 = property on="light_64" class="Bool (严格)"("Colors [4]"=w297) -> ()  [unwired: 2 in, 2 out]
            n883 = property on="light_65" class="Bool (严格)"("Colors [4]"=w297) -> ()  [unwired: 2 in, 2 out]
            n884 = property on="light_66" class="Bool (严格)"("Colors [4]"=w297) -> ()  [unwired: 2 in, 2 out]
            n885 = property on="light_67" class="Bool (严格)"("Colors [4]"=w297) -> ()  [unwired: 2 in, 2 out]
            n886 = property on="light_68" class="Bool (严格)"("Colors [4]"=w297) -> ()  [unwired: 2 in, 2 out]
            n887 = property on="light_69" class="Bool (严格)"("Colors [4]"=w297) -> ()  [unwired: 2 in, 2 out]
            n888 = property on="light_70" class="Bool (严格)"("Colors [4]"=w297) -> ()  [unwired: 2 in, 2 out]
            n889 = property on="light_71" class="Bool (严格)"("Colors [4]"=w297) -> ()  [unwired: 2 in, 2 out]
            n890 = property on="light_72" class="Bool (严格)"("Colors [4]"=w297) -> ()  [unwired: 2 in, 2 out]
            n891 = property on="light_73" class="Bool (严格)"("Colors [4]"=w297) -> ()  [unwired: 2 in, 2 out]
            n892 = property on="light_74" class="Bool (严格)"("Colors [4]"=w297) -> ()  [unwired: 2 in, 2 out]
            n893 = property on="light_75" class="Bool (严格)"("Colors [4]"=w297) -> ()  [unwired: 2 in, 2 out]
            n894 = property on="light_76" class="Bool (严格)"("Colors [4]"=w297) -> ()  [unwired: 2 in, 2 out]
            n895 = property on="light_77" class="Bool (严格)"("Colors [4]"=w297) -> ()  [unwired: 2 in, 2 out]
            n896 = property on="light_78" class="Bool (严格)"("Colors [4]"=w297) -> ()  [unwired: 2 in, 2 out]
            n897 = property on="light_79" class="Bool (严格)"("Colors [4]"=w297) -> ()  [unwired: 2 in, 2 out]
            n898 = property on="light_80" class="Bool (严格)"("Colors [4]"=w297) -> ()  [unwired: 2 in, 2 out]
            n899 = disable-structure shown="禁用" {
              frame Disabled {
                n900 = Initialize Array("", 16 ("维数大小"), 4 ("维数大小")) -> (w301:string[][])
                n901 = local write "D_IN_1"(w301) -> ()
                n902 = local write "D_IN_2"(w301) -> ()
                n903 = local write "D_IN_3"(w301) -> ()
                n904 = local write "D_IN_4"(w301) -> ()
                n905 = local write "D_IN_5"(w301) -> ()
              }
              frame Enabled {
              }
            }
            n906 = property on="btn_关闭" class="Bool"("DisabledEnum"=T1."Disabled and Grayed Out" ("禁用")) -> ()  [unwired: 2 in, 2 out]
          }
          frame #2 {
            w304 = 0 ("同步_A1")
            n907 = local read "数组_选择?"() -> (w310:bool[])
            n908 = Or Array Elements(Boolean array=w310) -> (logical OR=w309:bool)
            n909 = case shown="真" w309 {
              tunnel: w303 -> [_ w313]
              tunnel: w302 -> [_ w312]
              frame False {
                n910 = call "显示对话框信息"("Message"="请选择数字量输入路数") -> ()  [unwired: 9 in, 2 out]
              }
              frame True {
                n911 = Send Notification(notification="DInput" ("通知"), notifier=w313, error in (no error)=w312) -> ()  [unwired: 2 out]
              }
            }
            n912 = local write "第几组数据"(0 ("第几组数据")) -> ()
            n913 = local write "同步_A1"(w304) -> ()
            n914 = local write "同步_A2"(w304) -> ()
            n915 = Initialize Array(FALSE, 80 ("维数大小")) -> (w306:bool[])
            n916 = local write "合格？"(w306) -> ()
          }
        }
      }
      event "btn_全选": Value Change {
        w315 = TRUE ("单选_第41路")
        n917 = event-data() -> ()  [unwired: 1 in, 5 out]
        n918 = local write "单选_第1路"(w315) -> ()
        n919 = local write "单选_第2路"(w315) -> ()
        n920 = local write "单选_第3路"(w315) -> ()
        n921 = local write "单选_第4路"(w315) -> ()
        n922 = local write "单选_第5路"(w315) -> ()
        n923 = local write "单选_第6路"(w315) -> ()
        n924 = local write "单选_第7路"(w315) -> ()
        n925 = local write "单选_第8路"(w315) -> ()
        n926 = local write "单选_第9路"(w315) -> ()
        n927 = local write "单选_第10路"(w315) -> ()
        n928 = local write "单选_第11路"(w315) -> ()
        n929 = local write "单选_第12路"(w315) -> ()
        n930 = local write "单选_第13路"(w315) -> ()
        n931 = local write "单选_第14路"(w315) -> ()
        n932 = local write "单选_第15路"(w315) -> ()
        n933 = local write "单选_第16路"(w315) -> ()
        n934 = local write "单选_第17路"(w315) -> ()
        n935 = local write "单选_第18路"(w315) -> ()
        n936 = local write "单选_第19路"(w315) -> ()
        n937 = local write "单选_第20路"(w315) -> ()
        n938 = local write "单选_第21路"(w315) -> ()
        n939 = local write "单选_第22路"(w315) -> ()
        n940 = local write "单选_第23路"(w315) -> ()
        n941 = local write "单选_第24路"(w315) -> ()
        n942 = local write "单选_第25路"(w315) -> ()
        n943 = local write "单选_第26路"(w315) -> ()
        n944 = local write "单选_第27路"(w315) -> ()
        n945 = local write "单选_第28路"(w315) -> ()
        n946 = local write "单选_第29路"(w315) -> ()
        n947 = local write "单选_第30路"(w315) -> ()
        n948 = local write "单选_第31路"(w315) -> ()
        n949 = local write "单选_第32路"(w315) -> ()
        n950 = local write "单选_第33路"(w315) -> ()
        n951 = local write "单选_第34路"(w315) -> ()
        n952 = local write "单选_第35路"(w315) -> ()
        n953 = local write "单选_第36路"(w315) -> ()
        n954 = local write "单选_第37路"(w315) -> ()
        n955 = local write "单选_第38路"(w315) -> ()
        n956 = local write "单选_第39路"(w315) -> ()
        n957 = local write "单选_第40路"(w315) -> ()
        n958 = local write "单选_第41路"(w315) -> ()
        n959 = local write "单选_第42路"(w315) -> ()
        n960 = local write "单选_第43路"(w315) -> ()
        n961 = local write "单选_第44路"(w315) -> ()
        n962 = local write "单选_第45路"(w315) -> ()
        n963 = local write "单选_第46路"(w315) -> ()
        n964 = local write "单选_第47路"(w315) -> ()
        n965 = local write "单选_第48路"(w315) -> ()
        n966 = local write "单选_第49路"(w315) -> ()
        n967 = local write "单选_第50路"(w315) -> ()
        n968 = local write "单选_第51路"(w315) -> ()
        n969 = local write "单选_第52路"(w315) -> ()
        n970 = local write "单选_第53路"(w315) -> ()
        n971 = local write "单选_第54路"(w315) -> ()
        n972 = local write "单选_第55路"(w315) -> ()
        n973 = local write "单选_第56路"(w315) -> ()
        n974 = local write "单选_第57路"(w315) -> ()
        n975 = local write "单选_第58路"(w315) -> ()
        n976 = local write "单选_第59路"(w315) -> ()
        n977 = local write "单选_第60路"(w315) -> ()
        n978 = local write "单选_第61路"(w315) -> ()
        n979 = local write "单选_第62路"(w315) -> ()
        n980 = local write "单选_第63路"(w315) -> ()
        n981 = local write "单选_第64路"(w315) -> ()
        n982 = local write "单选_第71路"(w315) -> ()
        n983 = local write "单选_第79路"(w315) -> ()
        n984 = local write "单选_第65路"(w315) -> ()
        n985 = local write "单选_第66路"(w315) -> ()
        n986 = local write "单选_第67路"(w315) -> ()
        n987 = local write "单选_第68路"(w315) -> ()
        n988 = local write "单选_第69路"(w315) -> ()
        n989 = local write "单选_第70路"(w315) -> ()
        n990 = local write "单选_第72路"(w315) -> ()
        n991 = local write "单选_第73路"(w315) -> ()
        n992 = local write "单选_第74路"(w315) -> ()
        n993 = local write "单选_第75路"(w315) -> ()
        n994 = local write "单选_第76路"(w315) -> ()
        n995 = local write "单选_第77路"(w315) -> ()
        n996 = local write "单选_第78路"(w315) -> ()
        n997 = local write "单选_第80路"(w315) -> ()
      }
      event "btn_反选": Value Change {
        n998 = event-data() -> ()  [unwired: 1 in, 5 out]
        n999 = local read "单选_第1路"() -> (w475:bool)
        n1000 = local read "单选_第2路"() -> (w473:bool)
        n1001 = local read "单选_第3路"() -> (w471:bool)
        n1002 = local read "单选_第4路"() -> (w469:bool)
        n1003 = local read "单选_第5路"() -> (w467:bool)
        n1004 = local read "单选_第6路"() -> (w465:bool)
        n1005 = local read "单选_第7路"() -> (w464:bool)
        n1006 = local read "单选_第8路"() -> (w463:bool)
        n1007 = local read "单选_第9路"() -> (w462:bool)
        n1008 = local read "单选_第10路"() -> (w461:bool)
        n1009 = local read "单选_第11路"() -> (w460:bool)
        n1010 = local read "单选_第12路"() -> (w459:bool)
        n1011 = local read "单选_第13路"() -> (w458:bool)
        n1012 = local read "单选_第14路"() -> (w457:bool)
        n1013 = local read "单选_第15路"() -> (w456:bool)
        n1014 = local read "单选_第16路"() -> (w455:bool)
        n1015 = local read "单选_第17路"() -> (w454:bool)
        n1016 = local read "单选_第18路"() -> (w453:bool)
        n1017 = local read "单选_第19路"() -> (w452:bool)
        n1018 = local read "单选_第20路"() -> (w451:bool)
        n1019 = local read "单选_第21路"() -> (w450:bool)
        n1020 = local read "单选_第22路"() -> (w449:bool)
        n1021 = local read "单选_第23路"() -> (w448:bool)
        n1022 = local read "单选_第24路"() -> (w447:bool)
        n1023 = local read "单选_第25路"() -> (w446:bool)
        n1024 = local read "单选_第26路"() -> (w445:bool)
        n1025 = local read "单选_第27路"() -> (w444:bool)
        n1026 = local read "单选_第28路"() -> (w443:bool)
        n1027 = local read "单选_第29路"() -> (w442:bool)
        n1028 = local read "单选_第30路"() -> (w441:bool)
        n1029 = local read "单选_第31路"() -> (w440:bool)
        n1030 = local read "单选_第32路"() -> (w439:bool)
        n1031 = local read "单选_第33路"() -> (w438:bool)
        n1032 = local read "单选_第34路"() -> (w437:bool)
        n1033 = local read "单选_第35路"() -> (w436:bool)
        n1034 = local read "单选_第36路"() -> (w435:bool)
        n1035 = local read "单选_第37路"() -> (w434:bool)
        n1036 = local read "单选_第38路"() -> (w433:bool)
        n1037 = local read "单选_第39路"() -> (w432:bool)
        n1038 = local read "单选_第40路"() -> (w431:bool)
        n1039 = Not(x=w475) -> (.not. x?=w474:bool)
        n1040 = Not(x=w473) -> (.not. x?=w472:bool)
        n1041 = Not(x=w471) -> (.not. x?=w470:bool)
        n1042 = Not(x=w469) -> (.not. x?=w468:bool)
        n1043 = Not(x=w467) -> (.not. x?=w466:bool)
        n1044 = Not(x=w465) -> (.not. x?=w430:bool)
        n1045 = Not(x=w464) -> (.not. x?=w429:bool)
        n1046 = Not(x=w463) -> (.not. x?=w428:bool)
        n1047 = Not(x=w462) -> (.not. x?=w427:bool)
        n1048 = Not(x=w461) -> (.not. x?=w426:bool)
        n1049 = Not(x=w460) -> (.not. x?=w425:bool)
        n1050 = Not(x=w459) -> (.not. x?=w424:bool)
        n1051 = Not(x=w458) -> (.not. x?=w423:bool)
        n1052 = Not(x=w457) -> (.not. x?=w422:bool)
        n1053 = Not(x=w456) -> (.not. x?=w421:bool)
        n1054 = Not(x=w455) -> (.not. x?=w420:bool)
        n1055 = Not(x=w454) -> (.not. x?=w419:bool)
        n1056 = Not(x=w453) -> (.not. x?=w418:bool)
        n1057 = Not(x=w452) -> (.not. x?=w417:bool)
        n1058 = Not(x=w451) -> (.not. x?=w416:bool)
        n1059 = Not(x=w450) -> (.not. x?=w415:bool)
        n1060 = Not(x=w449) -> (.not. x?=w414:bool)
        n1061 = Not(x=w448) -> (.not. x?=w413:bool)
        n1062 = Not(x=w447) -> (.not. x?=w412:bool)
        n1063 = Not(x=w446) -> (.not. x?=w411:bool)
        n1064 = Not(x=w445) -> (.not. x?=w410:bool)
        n1065 = Not(x=w444) -> (.not. x?=w409:bool)
        n1066 = Not(x=w443) -> (.not. x?=w408:bool)
        n1067 = Not(x=w442) -> (.not. x?=w407:bool)
        n1068 = Not(x=w441) -> (.not. x?=w406:bool)
        n1069 = Not(x=w440) -> (.not. x?=w405:bool)
        n1070 = Not(x=w439) -> (.not. x?=w404:bool)
        n1071 = Not(x=w438) -> (.not. x?=w403:bool)
        n1072 = Not(x=w437) -> (.not. x?=w402:bool)
        n1073 = Not(x=w436) -> (.not. x?=w401:bool)
        n1074 = Not(x=w435) -> (.not. x?=w400:bool)
        n1075 = Not(x=w434) -> (.not. x?=w399:bool)
        n1076 = Not(x=w433) -> (.not. x?=w398:bool)
        n1077 = Not(x=w432) -> (.not. x?=w397:bool)
        n1078 = Not(x=w431) -> (.not. x?=w396:bool)
        n1079 = local write "单选_第1路"(w474) -> ()
        n1080 = local write "单选_第2路"(w472) -> ()
        n1081 = local write "单选_第3路"(w470) -> ()
        n1082 = local write "单选_第4路"(w468) -> ()
        n1083 = local write "单选_第5路"(w466) -> ()
        n1084 = local write "单选_第6路"(w430) -> ()
        n1085 = local write "单选_第7路"(w429) -> ()
        n1086 = local write "单选_第8路"(w428) -> ()
        n1087 = local write "单选_第9路"(w427) -> ()
        n1088 = local write "单选_第10路"(w426) -> ()
        n1089 = local write "单选_第11路"(w425) -> ()
        n1090 = local write "单选_第12路"(w424) -> ()
        n1091 = local write "单选_第13路"(w423) -> ()
        n1092 = local write "单选_第14路"(w422) -> ()
        n1093 = local write "单选_第15路"(w421) -> ()
        n1094 = local write "单选_第16路"(w420) -> ()
        n1095 = local write "单选_第17路"(w419) -> ()
        n1096 = local write "单选_第18路"(w418) -> ()
        n1097 = local write "单选_第19路"(w417) -> ()
        n1098 = local write "单选_第20路"(w416) -> ()
        n1099 = local write "单选_第21路"(w415) -> ()
        n1100 = local write "单选_第22路"(w414) -> ()
        n1101 = local write "单选_第23路"(w413) -> ()
        n1102 = local write "单选_第24路"(w412) -> ()
        n1103 = local write "单选_第25路"(w411) -> ()
        n1104 = local write "单选_第26路"(w410) -> ()
        n1105 = local write "单选_第27路"(w409) -> ()
        n1106 = local write "单选_第28路"(w408) -> ()
        n1107 = local write "单选_第29路"(w407) -> ()
        n1108 = local write "单选_第30路"(w406) -> ()
        n1109 = local write "单选_第31路"(w405) -> ()
        n1110 = local write "单选_第32路"(w404) -> ()
        n1111 = local write "单选_第33路"(w403) -> ()
        n1112 = local write "单选_第34路"(w402) -> ()
        n1113 = local write "单选_第35路"(w401) -> ()
        n1114 = local write "单选_第36路"(w400) -> ()
        n1115 = local write "单选_第37路"(w399) -> ()
        n1116 = local write "单选_第38路"(w398) -> ()
        n1117 = local write "单选_第39路"(w397) -> ()
        n1118 = local write "单选_第40路"(w396) -> ()
        n1119 = local read "单选_第71路"() -> (w365:bool)
        n1120 = local read "单选_第79路"() -> (w357:bool)
        n1121 = local read "单选_第41路"() -> (w395:bool)
        n1122 = local read "单选_第42路"() -> (w394:bool)
        n1123 = local read "单选_第43路"() -> (w393:bool)
        n1124 = local read "单选_第44路"() -> (w392:bool)
        n1125 = local read "单选_第45路"() -> (w391:bool)
        n1126 = local read "单选_第46路"() -> (w390:bool)
        n1127 = local read "单选_第47路"() -> (w389:bool)
        n1128 = local read "单选_第48路"() -> (w388:bool)
        n1129 = local read "单选_第49路"() -> (w387:bool)
        n1130 = local read "单选_第50路"() -> (w386:bool)
        n1131 = local read "单选_第51路"() -> (w385:bool)
        n1132 = local read "单选_第52路"() -> (w384:bool)
        n1133 = local read "单选_第53路"() -> (w383:bool)
        n1134 = local read "单选_第54路"() -> (w382:bool)
        n1135 = local read "单选_第55路"() -> (w381:bool)
        n1136 = local read "单选_第56路"() -> (w380:bool)
        n1137 = local read "单选_第57路"() -> (w379:bool)
        n1138 = local read "单选_第58路"() -> (w378:bool)
        n1139 = local read "单选_第59路"() -> (w377:bool)
        n1140 = local read "单选_第60路"() -> (w376:bool)
        n1141 = local read "单选_第61路"() -> (w375:bool)
        n1142 = local read "单选_第62路"() -> (w374:bool)
        n1143 = local read "单选_第63路"() -> (w373:bool)
        n1144 = local read "单选_第64路"() -> (w372:bool)
        n1145 = local read "单选_第65路"() -> (w371:bool)
        n1146 = local read "单选_第66路"() -> (w370:bool)
        n1147 = local read "单选_第67路"() -> (w369:bool)
        n1148 = local read "单选_第68路"() -> (w368:bool)
        n1149 = local read "单选_第69路"() -> (w367:bool)
        n1150 = local read "单选_第70路"() -> (w366:bool)
        n1151 = local read "单选_第72路"() -> (w364:bool)
        n1152 = local read "单选_第73路"() -> (w363:bool)
        n1153 = local read "单选_第74路"() -> (w362:bool)
        n1154 = local read "单选_第75路"() -> (w361:bool)
        n1155 = local read "单选_第76路"() -> (w360:bool)
        n1156 = local read "单选_第77路"() -> (w359:bool)
        n1157 = local read "单选_第78路"() -> (w358:bool)
        n1158 = local read "单选_第80路"() -> (w356:bool)
        n1159 = Not(x=w395) -> (.not. x?=w355:bool)
        n1160 = Not(x=w394) -> (.not. x?=w354:bool)
        n1161 = Not(x=w393) -> (.not. x?=w353:bool)
        n1162 = Not(x=w392) -> (.not. x?=w352:bool)
        n1163 = Not(x=w391) -> (.not. x?=w351:bool)
        n1164 = Not(x=w390) -> (.not. x?=w350:bool)
        n1165 = Not(x=w389) -> (.not. x?=w349:bool)
        n1166 = Not(x=w388) -> (.not. x?=w348:bool)
        n1167 = Not(x=w387) -> (.not. x?=w347:bool)
        n1168 = Not(x=w386) -> (.not. x?=w346:bool)
        n1169 = Not(x=w385) -> (.not. x?=w345:bool)
        n1170 = Not(x=w384) -> (.not. x?=w344:bool)
        n1171 = Not(x=w383) -> (.not. x?=w343:bool)
        n1172 = Not(x=w382) -> (.not. x?=w342:bool)
        n1173 = Not(x=w381) -> (.not. x?=w341:bool)
        n1174 = Not(x=w380) -> (.not. x?=w340:bool)
        n1175 = Not(x=w379) -> (.not. x?=w339:bool)
        n1176 = Not(x=w378) -> (.not. x?=w338:bool)
        n1177 = Not(x=w377) -> (.not. x?=w337:bool)
        n1178 = Not(x=w376) -> (.not. x?=w336:bool)
        n1179 = Not(x=w375) -> (.not. x?=w335:bool)
        n1180 = Not(x=w374) -> (.not. x?=w334:bool)
        n1181 = Not(x=w373) -> (.not. x?=w333:bool)
        n1182 = Not(x=w372) -> (.not. x?=w332:bool)
        n1183 = Not(x=w371) -> (.not. x?=w331:bool)
        n1184 = Not(x=w370) -> (.not. x?=w330:bool)
        n1185 = Not(x=w369) -> (.not. x?=w329:bool)
        n1186 = Not(x=w368) -> (.not. x?=w328:bool)
        n1187 = Not(x=w367) -> (.not. x?=w327:bool)
        n1188 = Not(x=w366) -> (.not. x?=w326:bool)
        n1189 = Not(x=w365) -> (.not. x?=w325:bool)
        n1190 = Not(x=w364) -> (.not. x?=w324:bool)
        n1191 = Not(x=w363) -> (.not. x?=w323:bool)
        n1192 = Not(x=w362) -> (.not. x?=w322:bool)
        n1193 = Not(x=w361) -> (.not. x?=w321:bool)
        n1194 = Not(x=w360) -> (.not. x?=w320:bool)
        n1195 = Not(x=w359) -> (.not. x?=w319:bool)
        n1196 = Not(x=w358) -> (.not. x?=w318:bool)
        n1197 = Not(x=w357) -> (.not. x?=w317:bool)
        n1198 = Not(x=w356) -> (.not. x?=w316:bool)
        n1199 = local write "单选_第71路"(w325) -> ()
        n1200 = local write "单选_第79路"(w317) -> ()
        n1201 = local write "单选_第41路"(w355) -> ()
        n1202 = local write "单选_第42路"(w354) -> ()
        n1203 = local write "单选_第43路"(w353) -> ()
        n1204 = local write "单选_第44路"(w352) -> ()
        n1205 = local write "单选_第45路"(w351) -> ()
        n1206 = local write "单选_第46路"(w350) -> ()
        n1207 = local write "单选_第47路"(w349) -> ()
        n1208 = local write "单选_第48路"(w348) -> ()
        n1209 = local write "单选_第49路"(w347) -> ()
        n1210 = local write "单选_第50路"(w346) -> ()
        n1211 = local write "单选_第51路"(w345) -> ()
        n1212 = local write "单选_第52路"(w344) -> ()
        n1213 = local write "单选_第53路"(w343) -> ()
        n1214 = local write "单选_第54路"(w342) -> ()
        n1215 = local write "单选_第55路"(w341) -> ()
        n1216 = local write "单选_第56路"(w340) -> ()
        n1217 = local write "单选_第57路"(w339) -> ()
        n1218 = local write "单选_第58路"(w338) -> ()
        n1219 = local write "单选_第59路"(w337) -> ()
        n1220 = local write "单选_第60路"(w336) -> ()
        n1221 = local write "单选_第61路"(w335) -> ()
        n1222 = local write "单选_第62路"(w334) -> ()
        n1223 = local write "单选_第63路"(w333) -> ()
        n1224 = local write "单选_第64路"(w332) -> ()
        n1225 = local write "单选_第65路"(w331) -> ()
        n1226 = local write "单选_第66路"(w330) -> ()
        n1227 = local write "单选_第67路"(w329) -> ()
        n1228 = local write "单选_第68路"(w328) -> ()
        n1229 = local write "单选_第69路"(w327) -> ()
        n1230 = local write "单选_第70路"(w326) -> ()
        n1231 = local write "单选_第72路"(w324) -> ()
        n1232 = local write "单选_第73路"(w323) -> ()
        n1233 = local write "单选_第74路"(w322) -> ()
        n1234 = local write "单选_第75路"(w321) -> ()
        n1235 = local write "单选_第76路"(w320) -> ()
        n1236 = local write "单选_第77路"(w319) -> ()
        n1237 = local write "单选_第78路"(w318) -> ()
        n1238 = local write "单选_第80路"(w316) -> ()
      }
      event "btn_置1": Value Change {
        w476 = enum16{"0", "1"}."1" ("输入值_41")
        n1239 = event-data() -> ()  [unwired: 1 in, 5 out]
        n1240 = local write "输入值_1"(w476) -> ()
        n1241 = local write "输入值_2"(w476) -> ()
        n1242 = local write "输入值_3"(w476) -> ()
        n1243 = local write "输入值_4"(w476) -> ()
        n1244 = local write "输入值_5"(w476) -> ()
        n1245 = local write "输入值_6"(w476) -> ()
        n1246 = local write "输入值_7"(w476) -> ()
        n1247 = local write "输入值_8"(w476) -> ()
        n1248 = local write "输入值_9"(w476) -> ()
        n1249 = local write "输入值_10"(w476) -> ()
        n1250 = local write "输入值_11"(w476) -> ()
        n1251 = local write "输入值_12"(w476) -> ()
        n1252 = local write "输入值_13"(w476) -> ()
        n1253 = local write "输入值_14"(w476) -> ()
        n1254 = local write "输入值_15"(w476) -> ()
        n1255 = local write "输入值_16"(w476) -> ()
        n1256 = local write "输入值_17"(w476) -> ()
        n1257 = local write "输入值_18"(w476) -> ()
        n1258 = local write "输入值_19"(w476) -> ()
        n1259 = local write "输入值_20"(w476) -> ()
        n1260 = local write "输入值_21"(w476) -> ()
        n1261 = local write "输入值_22"(w476) -> ()
        n1262 = local write "输入值_23"(w476) -> ()
        n1263 = local write "输入值_24"(w476) -> ()
        n1264 = local write "输入值_25"(w476) -> ()
        n1265 = local write "输入值_26"(w476) -> ()
        n1266 = local write "输入值_27"(w476) -> ()
        n1267 = local write "输入值_28"(w476) -> ()
        n1268 = local write "输入值_29"(w476) -> ()
        n1269 = local write "输入值_30"(w476) -> ()
        n1270 = local write "输入值_31"(w476) -> ()
        n1271 = local write "输入值_32"(w476) -> ()
        n1272 = local write "输入值_33"(w476) -> ()
        n1273 = local write "输入值_34"(w476) -> ()
        n1274 = local write "输入值_35"(w476) -> ()
        n1275 = local write "输入值_36"(w476) -> ()
        n1276 = local write "输入值_37"(w476) -> ()
        n1277 = local write "输入值_38"(w476) -> ()
        n1278 = local write "输入值_39"(w476) -> ()
        n1279 = local write "输入值_40"(w476) -> ()
        n1280 = local write "输入值_41"(w476) -> ()
        n1281 = local write "输入值_42"(w476) -> ()
        n1282 = local write "输入值_43"(w476) -> ()
        n1283 = local write "输入值_44"(w476) -> ()
        n1284 = local write "输入值_45"(w476) -> ()
        n1285 = local write "输入值_46"(w476) -> ()
        n1286 = local write "输入值_47"(w476) -> ()
        n1287 = local write "输入值_48"(w476) -> ()
        n1288 = local write "输入值_49"(w476) -> ()
        n1289 = local write "输入值_50"(w476) -> ()
        n1290 = local write "输入值_51"(w476) -> ()
        n1291 = local write "输入值_52"(w476) -> ()
        n1292 = local write "输入值_53"(w476) -> ()
        n1293 = local write "输入值_54"(w476) -> ()
        n1294 = local write "输入值_55"(w476) -> ()
        n1295 = local write "输入值_56"(w476) -> ()
        n1296 = local write "输入值_57"(w476) -> ()
        n1297 = local write "输入值_58"(w476) -> ()
        n1298 = local write "输入值_59"(w476) -> ()
        n1299 = local write "输入值_60"(w476) -> ()
        n1300 = local write "输入值_61"(w476) -> ()
        n1301 = local write "输入值_62"(w476) -> ()
        n1302 = local write "输入值_63"(w476) -> ()
        n1303 = local write "输入值_64"(w476) -> ()
        n1304 = local write "输入值_65"(w476) -> ()
        n1305 = local write "输入值_66"(w476) -> ()
        n1306 = local write "输入值_67"(w476) -> ()
        n1307 = local write "输入值_68"(w476) -> ()
        n1308 = local write "输入值_69"(w476) -> ()
        n1309 = local write "输入值_70"(w476) -> ()
        n1310 = local write "输入值_71"(w476) -> ()
        n1311 = local write "输入值_72"(w476) -> ()
        n1312 = local write "输入值_73"(w476) -> ()
        n1313 = local write "输入值_74"(w476) -> ()
        n1314 = local write "输入值_75"(w476) -> ()
        n1315 = local write "输入值_76"(w476) -> ()
        n1316 = local write "输入值_77"(w476) -> ()
        n1317 = local write "输入值_78"(w476) -> ()
        n1318 = local write "输入值_79"(w476) -> ()
        n1319 = local write "输入值_80"(w476) -> ()
      }
      event "btn_置0": Value Change {
        w477 = enum16{"0", "1"}."0" ("输入值_41")
        n1320 = event-data() -> ()  [unwired: 1 in, 5 out]
        n1321 = local write "输入值_1"(w477) -> ()
        n1322 = local write "输入值_2"(w477) -> ()
        n1323 = local write "输入值_3"(w477) -> ()
        n1324 = local write "输入值_4"(w477) -> ()
        n1325 = local write "输入值_5"(w477) -> ()
        n1326 = local write "输入值_6"(w477) -> ()
        n1327 = local write "输入值_7"(w477) -> ()
        n1328 = local write "输入值_8"(w477) -> ()
        n1329 = local write "输入值_9"(w477) -> ()
        n1330 = local write "输入值_10"(w477) -> ()
        n1331 = local write "输入值_11"(w477) -> ()
        n1332 = local write "输入值_12"(w477) -> ()
        n1333 = local write "输入值_13"(w477) -> ()
        n1334 = local write "输入值_14"(w477) -> ()
        n1335 = local write "输入值_15"(w477) -> ()
        n1336 = local write "输入值_16"(w477) -> ()
        n1337 = local write "输入值_17"(w477) -> ()
        n1338 = local write "输入值_18"(w477) -> ()
        n1339 = local write "输入值_19"(w477) -> ()
        n1340 = local write "输入值_20"(w477) -> ()
        n1341 = local write "输入值_21"(w477) -> ()
        n1342 = local write "输入值_22"(w477) -> ()
        n1343 = local write "输入值_23"(w477) -> ()
        n1344 = local write "输入值_24"(w477) -> ()
        n1345 = local write "输入值_25"(w477) -> ()
        n1346 = local write "输入值_26"(w477) -> ()
        n1347 = local write "输入值_27"(w477) -> ()
        n1348 = local write "输入值_28"(w477) -> ()
        n1349 = local write "输入值_29"(w477) -> ()
        n1350 = local write "输入值_30"(w477) -> ()
        n1351 = local write "输入值_31"(w477) -> ()
        n1352 = local write "输入值_32"(w477) -> ()
        n1353 = local write "输入值_33"(w477) -> ()
        n1354 = local write "输入值_34"(w477) -> ()
        n1355 = local write "输入值_35"(w477) -> ()
        n1356 = local write "输入值_36"(w477) -> ()
        n1357 = local write "输入值_37"(w477) -> ()
        n1358 = local write "输入值_38"(w477) -> ()
        n1359 = local write "输入值_39"(w477) -> ()
        n1360 = local write "输入值_40"(w477) -> ()
        n1361 = local write "输入值_41"(w477) -> ()
        n1362 = local write "输入值_42"(w477) -> ()
        n1363 = local write "输入值_43"(w477) -> ()
        n1364 = local write "输入值_44"(w477) -> ()
        n1365 = local write "输入值_45"(w477) -> ()
        n1366 = local write "输入值_46"(w477) -> ()
        n1367 = local write "输入值_47"(w477) -> ()
        n1368 = local write "输入值_48"(w477) -> ()
        n1369 = local write "输入值_49"(w477) -> ()
        n1370 = local write "输入值_50"(w477) -> ()
        n1371 = local write "输入值_51"(w477) -> ()
        n1372 = local write "输入值_52"(w477) -> ()
        n1373 = local write "输入值_53"(w477) -> ()
        n1374 = local write "输入值_54"(w477) -> ()
        n1375 = local write "输入值_55"(w477) -> ()
        n1376 = local write "输入值_56"(w477) -> ()
        n1377 = local write "输入值_57"(w477) -> ()
        n1378 = local write "输入值_58"(w477) -> ()
        n1379 = local write "输入值_59"(w477) -> ()
        n1380 = local write "输入值_60"(w477) -> ()
        n1381 = local write "输入值_61"(w477) -> ()
        n1382 = local write "输入值_62"(w477) -> ()
        n1383 = local write "输入值_63"(w477) -> ()
        n1384 = local write "输入值_64"(w477) -> ()
        n1385 = local write "输入值_65"(w477) -> ()
        n1386 = local write "输入值_66"(w477) -> ()
        n1387 = local write "输入值_67"(w477) -> ()
        n1388 = local write "输入值_68"(w477) -> ()
        n1389 = local write "输入值_69"(w477) -> ()
        n1390 = local write "输入值_70"(w477) -> ()
        n1391 = local write "输入值_71"(w477) -> ()
        n1392 = local write "输入值_72"(w477) -> ()
        n1393 = local write "输入值_73"(w477) -> ()
        n1394 = local write "输入值_74"(w477) -> ()
        n1395 = local write "输入值_75"(w477) -> ()
        n1396 = local write "输入值_76"(w477) -> ()
        n1397 = local write "输入值_77"(w477) -> ()
        n1398 = local write "输入值_78"(w477) -> ()
        n1399 = local write "输入值_79"(w477) -> ()
        n1400 = local write "输入值_80"(w477) -> ()
      }
    }
  }
  n1401 = disable-structure shown="禁用" {
    frame Disabled {
      n1402 = for {
        N: 16 -> [_]
        i -> [w480]
        n1403 = for {
          N: 4 -> [_]
          tunnel: w480 -> [w484]
          i -> [w485]
          w482 = u32 24 ("活动单元格:单元格大小:高度")
          n1404 = Bundle(w484, w485) -> (w483:cluster{i32, i32})  [unwired: 1 in]
          n1405 = property on="D_IN_1" class="Tbl (严格)"("Active Cell"=w483) -> (error out=w486:errorcluster)  [unwired: 2 in, 1 out]
          n1406 = property on="D_IN_2" class="Tbl (严格)"("Active Cell"=w483) -> ()  [unwired: 2 in, 2 out]
          n1407 = property on="D_IN_3" class="Tbl (严格)"("Active Cell"=w483) -> ()  [unwired: 2 in, 2 out]
          n1408 = property on="D_IN_4" class="Tbl (严格)"("Active Cell"=w483) -> ()  [unwired: 2 in, 2 out]
          n1409 = property on="D_IN_5" class="Tbl (严格)"("Active Cell"=w483) -> ()  [unwired: 2 in, 2 out]
          n1410 = property on="D_IN_1" class="Tbl (严格)"(error in=w486, "Height"=w482) -> ()  [unwired: 1 in, 2 out]
          n1411 = property on="D_IN_2" class="Tbl (严格)"("Height"=w482) -> ()  [unwired: 2 in, 2 out]
          n1412 = property on="D_IN_3" class="Tbl (严格)"("Height"=w482) -> ()  [unwired: 2 in, 2 out]
          n1413 = property on="D_IN_4" class="Tbl (严格)"("Height"=w482) -> ()  [unwired: 2 in, 2 out]
          n1414 = property on="D_IN_5" class="Tbl (严格)"("Height"=w482) -> ()  [unwired: 2 in, 2 out]
        }
        n1415 = Wait Until Next ms Multiple(millisecond multiple=u32 10 ("毫秒倍数")) -> ()  [unwired: 1 out]
      }
    }
    frame Enabled {
    }
  }
  n1416 = Obtain Notifier(name (unnamed)=w8, notification data type=w8) -> (notifier out=w16:refnum<notifier>, error out=w15:errorcluster)  [unwired: 2 in, 1 out]
  n1417 = disable-structure shown="启用" {
    frame Disabled {
      n1418 = for {
        N: 40 -> [_]
        i -> [w492]
        n1419 = Wait Until Next ms Multiple(millisecond multiple=u32 10 ("毫秒倍数")) -> ()  [unwired: 1 out]
        n1420 = Bundle(w492, "y"=-1) -> (w491:cluster{i32, "y":i32})  [unwired: 1 in]
        n1421 = property on="D_IN_1" class="Tbl (严格)"("Active Cell"=w491) -> (error out=w490:errorcluster)  [unwired: 2 in, 1 out]
        n1422 = property on="D_IN_1" class="Tbl (严格)"(error in=w490, "Cell BG Color"=u32 12369084) -> ()  [unwired: 1 in, 2 out]
      }
    }
    frame Enabled {
    }
  }
  n1423 = disable-structure shown="启用" {
    frame Disabled {
      n1424 = for {
        N: 40 -> [_]
        i -> [w496]
        n1425 = for {
          N: 4 -> [_]
          tunnel: w496 -> [w504]
          i -> [w501]
          n1426 = Bundle(w504, w501) -> (w500:cluster{i32, i32})  [unwired: 1 in]
          n1427 = Quotient & Remainder(x=w504, y=2) -> (x-y*floor(x/y)=w502:i32)  [unwired: 1 out]
          n1428 = property on="D_IN_1" class="Tbl (严格)"("Active Cell"=w500) -> (error out=w498:errorcluster)  [unwired: 2 in, 1 out]
          n1429 = Equal To 0?(x=w502) -> (x = 0?=w505:bool)
          n1430 = case shown="真" w505 {
            tunnel: [u32 16448250 u32 15723488] -> w499
            frame False {
            }
            frame True {
            }
          }
          n1431 = property on="D_IN_1" class="Tbl (严格)"(error in=w498, "Cell BG Color"=w499) -> ()  [unwired: 1 in, 2 out]
        }
        n1432 = Wait Until Next ms Multiple(millisecond multiple=u32 10 ("毫秒倍数")) -> ()  [unwired: 1 out]
      }
    }
    frame Enabled {
    }
  }
  n1433 = Obtain Notifier(name (unnamed)=w4, notification data type=w4) -> (notifier out=w3:refnum<notifier>, error out=w2:errorcluster)  [unwired: 2 in, 1 out]
  n1434 = while {
    tunnel: w16 -> [w514]
    tunnel: w15 -> [w513]
    tunnel: [w512] -> w14
    tunnel: [w511] -> w13
    tunnel: w3 -> [w509]
    tunnel: w2 -> [w508]
    stop <- w515 stop-if-true
    n1435 = Wait Until Next ms Multiple(millisecond multiple=u32 20 ("毫秒倍数")) -> ()  [unwired: 1 out]
    n1436 = Wait on Notification(notifier=w514, timeout in ms (-1)=20 ("超时毫秒(-1)"), error in (no error)=w513) -> (notifier out=w512:refnum<notifier>, notification=w519:string, error out=w511:errorcluster)  [unwired: 1 in, 1 out]
    n1437 = Equal?(x=w519, y="DInput" ("通知")) -> (x = y?=w510:bool)
    n1438 = case shown="真" w510 {
      tunnel: w509 -> [_ w521]
      tunnel: w508 -> [_ w520]
      frame False {
      }
      frame True {
        n1439 = stacked-sequence {
          tunnel: w521 -> [w523 _]
          tunnel: w520 -> [w522 _]
          frame #0 {
            n1440 = for {
              N: 80 -> [_]
              tunnel: w523 -> [w526]
              tunnel: w522 -> [w525]
              i -> [w528]
              n1441 = local read "数组_选择?"() -> (w530:bool[])
              n1442 = local read "数组_输入值"() -> (w527:enum16{"0", "1"}[])
              n1443 = Index Array(array=w530, index=w528) -> (element=w529:bool)
              n1444 = case shown="真" w529 {
                tunnel: w528 -> [_ w534]
                tunnel: w527 -> [_ w533]
                tunnel: w526 -> [_ w532]
                tunnel: w525 -> [_ w531]
                frame False {
                }
                frame True {
                  n1445 = case shown="真" TRUE {
                    tunnel: w534 -> [_ w539]
                    tunnel: w533 -> [_ w538]
                    tunnel: w532 -> [_ w537]
                    tunnel: w531 -> [_ w536]
                    frame False {
                    }
                    frame True {
                      n1446 = while {
                        tunnel: w539 -> [w546]
                        tunnel: w538 -> [w545]
                        tunnel: w537 -> [w541]
                        tunnel: w536 -> [w540]
                        stop <- w544 stop-if-true
                        n1447 = local read "同步_A1"() -> (w542:i32)
                        n1448 = Wait Until Next ms Multiple(millisecond multiple=u32 10 ("毫秒倍数")) -> ()  [unwired: 1 out]
                        n1449 = Equal?(x=w542, y=0) -> (x = y?=w547:bool)
                        n1450 = case shown="真" w547 {
                          tunnel: w546 -> [_ w554]
                          tunnel: w545 -> [_ w553]
                          tunnel: [FALSE w552] -> w544
                          tunnel: w541 -> [_ w551]
                          tunnel: w540 -> [_ w550]
                          frame False {
                          }
                          frame True {
                            n1451 = stacked-sequence {
                              tunnel: w554 -> [_ w566 _ _]
                              tunnel: w553 -> [_ w565 _ _]
                              tunnel: [_ _ _ w624] -> w552
                              tunnel: w551 -> [_ _ w621 _]
                              tunnel: w550 -> [_ _ w620 _]
                              frame #0 {
                                n1452 = Wait (ms)(milliseconds to wait=u32 100) -> ()  [unwired: 1 out]
                              }
                              frame #1 {
                                n1453 = To Long Integer(number=w566) -> (32bit integer=w556:i32)
                                n1454 = global read "试验配置信息.vi" "设定输出通道"() -> (w567:i32[])
                                n1455 = Index Array(array=w565, index=w556) -> (element=w563:enum16{"0", "1"})
                                n1456 = local write "第几组数据"(w556) -> ()
                                n1457 = Index Array(array=w567, index=w556) -> (element=w564:i32)
                                n1458 = case shown="0, 默认" w564 {
                                tunnel: w563 -> [w574 w577 w579 w582 w585 w588 w591 w594 w597 w600 w603 w606 w609 w612 w615 w618]
                                tunnel: [w573 w576 w580 w583 w586 w589 w592 w595 w598 w601 w604 w607 w610 w613 w616 w619] -> w557
                                frame 0, Default {
                                w572 = 0 ("y")
                                n1459 = Build Array(w574, w572, w572, w572, w572, w572, w572, w572, w572, w572, w572, w572, w572, w572, w572, w572) -> (w573:i32[])
                                }
                                frame 1 {
                                w575 = 0 ("y")
                                n1460 = Build Array(w575, w577, w575, w575, w575, w575, w575, w575, w575, w575, w575, w575, w575, w575, w575, w575) -> (w576:i32[])
                                }
                                frame 2 {
                                w578 = 0 ("y")
                                n1461 = Build Array(w578, w578, w579, w578, w578, w578, w578, w578, w578, w578, w578, w578, w578, w578, w578, w578) -> (w580:i32[])
                                }
                                frame 3 {
                                w581 = 0 ("y")
                                n1462 = Build Array(w581, w581, w581, w582, w581, w581, w581, w581, w581, w581, w581, w581, w581, w581, w581, w581) -> (w583:i32[])
                                }
                                frame 4 {
                                w584 = 0 ("y")
                                n1463 = Build Array(w584, w584, w584, w584, w585, w584, w584, w584, w584, w584, w584, w584, w584, w584, w584, w584) -> (w586:i32[])
                                }
                                frame 5 {
                                w587 = 0 ("y")
                                n1464 = Build Array(w587, w587, w587, w587, w587, w588, w587, w587, w587, w587, w587, w587, w587, w587, w587, w587) -> (w589:i32[])
                                }
                                frame 6 {
                                w590 = 0 ("y")
                                n1465 = Build Array(w590, w590, w590, w590, w590, w590, w591, w590, w590, w590, w590, w590, w590, w590, w590, w590) -> (w592:i32[])
                                }
                                frame 7 {
                                w593 = 0 ("y")
                                n1466 = Build Array(w593, w593, w593, w593, w593, w593, w593, w594, w593, w593, w593, w593, w593, w593, w593, w593) -> (w595:i32[])
                                }
                                frame 8 {
                                w596 = 0 ("y")
                                n1467 = Build Array(w596, w596, w596, w596, w596, w596, w596, w596, w597, w596, w596, w596, w596, w596, w596, w596) -> (w598:i32[])
                                }
                                frame 9 {
                                w599 = 0 ("y")
                                n1468 = Build Array(w599, w599, w599, w599, w599, w599, w599, w599, w599, w600, w599, w599, w599, w599, w599, w599) -> (w601:i32[])
                                }
                                frame 10 {
                                w602 = 0 ("y")
                                n1469 = Build Array(w602, w602, w602, w602, w602, w602, w602, w602, w602, w602, w603, w602, w602, w602, w602, w602) -> (w604:i32[])
                                }
                                frame 11 {
                                w605 = 0 ("y")
                                n1470 = Build Array(w605, w605, w605, w605, w605, w605, w605, w605, w605, w605, w605, w606, w605, w605, w605, w605) -> (w607:i32[])
                                }
                                frame 12 {
                                w608 = 0 ("y")
                                n1471 = Build Array(w608, w608, w608, w608, w608, w608, w608, w608, w608, w608, w608, w608, w609, w608, w608, w608) -> (w610:i32[])
                                }
                                frame 13 {
                                w611 = 0 ("y")
                                n1472 = Build Array(w611, w611, w611, w611, w611, w611, w611, w611, w611, w611, w611, w611, w611, w612, w611, w611) -> (w613:i32[])
                                }
                                frame 14 {
                                w614 = 0 ("y")
                                n1473 = Build Array(w614, w614, w614, w614, w614, w614, w614, w614, w614, w614, w614, w614, w614, w614, w615, w614) -> (w616:i32[])
                                }
                                frame 15 {
                                w617 = 0 ("y")
                                n1474 = Build Array(w617, w617, w617, w617, w617, w617, w617, w617, w617, w617, w617, w617, w617, w617, w617, w618) -> (w619:i32[])
                                }
                                }
                                n1475 = for {
                                tunnel: w557 -> [w569] mode=indexing
                                tunnel: [w568] -> w562 mode=indexing
                                n1476 = case shown="1" w569 {
                                tunnel: [FALSE TRUE] -> w568
                                frame 0, Default {
                                }
                                frame 1 {
                                }
                                }
                                }
                                n1477 = Boolean Array To Number ("布尔数组至数值转换")(Boolean array=w562) -> (number=w561:u16)
                                n1478 = Split Number(x=w561) -> (hi(x)=w558:u8, lo(x)=w559:u8)
                                n1479 = Build Array(w559, w558) -> (w560:u8[])
                                n1480 = call "DO"("dataIn(U8Array)"=w560) -> ()  [unwired: 2 in, 17 out]
                              }
                              frame #2 {
                                n1481 = local write "同步_A1"(1 ("同步_A1")) -> ()
                                n1482 = Send Notification(notification="DICheck" ("通知"), notifier=w621, error in (no error)=w620) -> ()  [unwired: 2 out]
                              }
                              frame #3 {
                                n1483 = local read "同步_A1"() -> (w625:i32)
                                n1484 = Equal?(x=w625, y=1) -> (x = y?=w624:bool)
                              }
                            }
                          }
                        }
                      }
                    }
                  }
                }
              }
            }
          }
          frame #1 {
            n1485 = property on="btn_关闭" class="Bool"("DisabledEnum"=T1."Enabled" ("禁用")) -> ()  [unwired: 2 in, 2 out]
          }
        }
      }
    }
    n1486 = local read "关闭？"() -> (w515:bool)
  }
  n1487 = Release Notifier(notifier=w14, error in (no error)=w13) -> ()  [unwired: 1 in, 3 out]
  n1488 = Obtain Notifier(name (unnamed)=w7, notification data type=w7) -> (notifier out=w12:refnum<notifier>, error out=w11:errorcluster)  [unwired: 2 in, 1 out]
  n1489 = while {
    tunnel: w12 -> [w632]
    tunnel: w11 -> [w631]
    tunnel: [w630] -> w10
    tunnel: [w629] -> w9
    stop <- w634 stop-if-true
    n1490 = Wait Until Next ms Multiple(millisecond multiple=u32 20 ("毫秒倍数")) -> ()  [unwired: 1 out]
    n1491 = Wait on Notification(notifier=w632, timeout in ms (-1)=20 ("超时毫秒(-1)"), error in (no error)=w631) -> (notifier out=w630:refnum<notifier>, notification=w635:string, error out=w629:errorcluster)  [unwired: 1 in, 1 out]
    n1492 = Equal?(x=w635, y="DICheck" ("通知")) -> (x = y?=w633:bool)
    n1493 = case shown="真" w633 {
      frame False {
      }
      frame True {
        n1494 = stacked-sequence {
          frame #0 {
            n1495 = local read "数组_输入值"() -> (w655:enum16{"0", "1"}[])
            n1496 = local read "第几组数据"() -> (w652:i32)
            n1497 = global read "试验配置信息.vi" "跳变方向"() -> (w657:i32[])
            n1498 = global read "试验配置信息.vi" "设定输入通道"() -> (w666:i32[])
            n1499 = Index Array(array=w655, index=w652) -> (element=w654:enum16{"0", "1"})
            n1500 = Index Array(array=w666, index=w652) -> (element=w639:i32)
            n1501 = Index Array(array=w657, index=w652) -> (element=w658:i32)
            n1502 = To Word Integer ("转换为双字节整型")(number=w654) -> (16bit integer=w656:i16)
            n1503 = call "DAQNavi Assistant"() -> ("dataOut(U8Array)"=w665:u8[])  [unwired: 2 in, 17 out]
            n1504 = Equal To 0?(x=w658) -> (x = 0?=w659:bool)
            n1505 = Not Equal To 0?(x=w656) -> (x != 0?=w660:bool)
            n1506 = Index Array(array=w665, index #1=0 ("索引"), index #2=1 ("索引")) -> (element #1=w643:u8, element #2=w642:u8)
            n1507 = case shown="真" w659 {
              tunnel: w660 -> [w780 w781]
              tunnel: [w779 w781] -> w661
              frame False {
                n1508 = Not(x=w780) -> (.not. x?=w779:bool)
              }
              frame True {
              }
            }
            n1509 = Number To Boolean Array(number=w643) -> (Boolean array=w647:bool[])
            n1510 = Number To Boolean Array(number=w642) -> (Boolean array=w646:bool[])
            n1511 = Build Array (concatenate)(w647, w646) -> (w641:bool[])
            n1512 = Boolean To (0,1)(Boolean=w661) -> (0, 1=w662:i16)
            n1513 = Boolean To (0,1) ("布尔值至(0,1)转换")(Boolean=w641) -> (0, 1=w640:i16[])
            n1514 = Index Array(array=w640, index=w639) -> (element=w638:i16)
            n1515 = Equal?(x=w638, y=w662) -> (x = y?=w663:bool)
            n1516 = Equal To 0?(x=w638) -> (x = 0?=w664:bool)
            n1517 = case shown="真" w664 {
              tunnel: ["1" "0"] -> w653
              frame False {
              }
              frame True {
              }
            }
            n1518 = case shown="假" w663 {
              tunnel: [cluster{u32, u32}[] [{16711680, 16711680}] ("结果") cluster{u32, u32}[] [{6618880, 6618880}] ("结果")] -> w648
              frame False {
              }
              frame True {
              }
            }
            n1519 = Quotient & Remainder(x=w652, y=16) -> (x-y*floor(x/y)=w649:i32, floor(x/y)=w650:i32)
            n1520 = case shown="0, 默认" w650 {
              tunnel: w648 -> [w667 w689 w711 w733 w755]
              tunnel: w653 -> [w669 w692 w714 w735 w757]
              tunnel: w649 -> [w668 w690 w712 w734 w756]
              frame 0, Default {
                n1521 = local read "D_IN_1"() -> (w672:string[][])
                n1522 = Replace Array Subset(array=w672, new element=w669, index (row)=w668, index (col)=2 ("禁用的索引 (列)")) -> (w670:string[][])
                n1523 = case shown="15" w668 {
                  tunnel: w667 -> [w673 w674 w675 w676 w677 w678 w679 w680 w681 w682 w683 w684 w685 w686 w687 w688]
                  frame 0, Default {
                    n1524 = property on="light_1" class="Bool (严格)"("Colors [4]"=w673) -> ()  [unwired: 2 in, 2 out]
                  }
                  frame 1 {
                    n1525 = property on="light_2" class="Bool (严格)"("Colors [4]"=w674) -> ()  [unwired: 2 in, 2 out]
                  }
                  frame 3 {
                    n1526 = property on="light_4" class="Bool (严格)"("Colors [4]"=w675) -> ()  [unwired: 2 in, 2 out]
                  }
                  frame 4 {
                    n1527 = property on="light_5" class="Bool (严格)"("Colors [4]"=w676) -> ()  [unwired: 2 in, 2 out]
                  }
                  frame 5 {
                    n1528 = property on="light_6" class="Bool (严格)"("Colors [4]"=w677) -> ()  [unwired: 2 in, 2 out]
                  }
                  frame 6 {
                    n1529 = property on="light_7" class="Bool (严格)"("Colors [4]"=w678) -> ()  [unwired: 2 in, 2 out]
                  }
                  frame 7 {
                    n1530 = property on="light_8" class="Bool (严格)"("Colors [4]"=w679) -> ()  [unwired: 2 in, 2 out]
                  }
                  frame 8 {
                    n1531 = property on="light_9" class="Bool (严格)"("Colors [4]"=w680) -> ()  [unwired: 2 in, 2 out]
                  }
                  frame 9 {
                    n1532 = property on="light_10" class="Bool (严格)"("Colors [4]"=w681) -> ()  [unwired: 2 in, 2 out]
                  }
                  frame 10 {
                    n1533 = property on="light_11" class="Bool (严格)"("Colors [4]"=w682) -> ()  [unwired: 2 in, 2 out]
                  }
                  frame 11 {
                    n1534 = property on="light_12" class="Bool (严格)"("Colors [4]"=w683) -> ()  [unwired: 2 in, 2 out]
                  }
                  frame 12 {
                    n1535 = property on="light_13" class="Bool (严格)"("Colors [4]"=w684) -> ()  [unwired: 2 in, 2 out]
                  }
                  frame 13 {
                    n1536 = property on="light_14" class="Bool (严格)"("Colors [4]"=w685) -> ()  [unwired: 2 in, 2 out]
                  }
                  frame 14 {
                    n1537 = property on="light_15" class="Bool (严格)"("Colors [4]"=w686) -> ()  [unwired: 2 in, 2 out]
                  }
                  frame 15 {
                    n1538 = property on="light_16" class="Bool (严格)"("Colors [4]"=w687) -> ()  [unwired: 2 in, 2 out]
                  }
                  frame 2 {
                    n1539 = property on="light_3" class="Bool (严格)"("Colors [4]"=w688) -> ()  [unwired: 2 in, 2 out]
                  }
                }
                n1540 = local write "D_IN_1"(w670) -> ()
              }
              frame 2 {
                n1541 = local read "D_IN_3"() -> (w693:string[][])
                n1542 = case shown="15" w690 {
                  tunnel: w689 -> [w695 w696 w697 w698 w699 w700 w701 w702 w703 w704 w705 w706 w707 w708 w709 w710]
                  frame 0, Default {
                    n1543 = property on="light_33" class="Bool (严格)"("Colors [4]"=w695) -> ()  [unwired: 2 in, 2 out]
                  }
                  frame 1 {
                    n1544 = property on="light_34" class="Bool (严格)"("Colors [4]"=w696) -> ()  [unwired: 2 in, 2 out]
                  }
                  frame 2 {
                    n1545 = property on="light_35" class="Bool (严格)"("Colors [4]"=w697) -> ()  [unwired: 2 in, 2 out]
                  }
                  frame 3 {
                    n1546 = property on="light_36" class="Bool (严格)"("Colors [4]"=w698) -> ()  [unwired: 2 in, 2 out]
                  }
                  frame 4 {
                    n1547 = property on="light_37" class="Bool (严格)"("Colors [4]"=w699) -> ()  [unwired: 2 in, 2 out]
                  }
                  frame 5 {
                    n1548 = property on="light_38" class="Bool (严格)"("Colors [4]"=w700) -> ()  [unwired: 2 in, 2 out]
                  }
                  frame 6 {
                    n1549 = property on="light_39" class="Bool (严格)"("Colors [4]"=w701) -> ()  [unwired: 2 in, 2 out]
                  }
                  frame 7 {
                    n1550 = property on="light_40" class="Bool (严格)"("Colors [4]"=w702) -> ()  [unwired: 2 in, 2 out]
                  }
                  frame 8 {
                    n1551 = property on="light_41" class="Bool (严格)"("Colors [4]"=w703) -> ()  [unwired: 2 in, 2 out]
                  }
                  frame 9 {
                    n1552 = property on="light_42" class="Bool (严格)"("Colors [4]"=w704) -> ()  [unwired: 2 in, 2 out]
                  }
                  frame 10 {
                    n1553 = property on="light_43" class="Bool (严格)"("Colors [4]"=w705) -> ()  [unwired: 2 in, 2 out]
                  }
                  frame 11 {
                    n1554 = property on="light_44" class="Bool (严格)"("Colors [4]"=w706) -> ()  [unwired: 2 in, 2 out]
                  }
                  frame 12 {
                    n1555 = property on="light_45" class="Bool (严格)"("Colors [4]"=w707) -> ()  [unwired: 2 in, 2 out]
                  }
                  frame 13 {
                    n1556 = property on="light_46" class="Bool (严格)"("Colors [4]"=w708) -> ()  [unwired: 2 in, 2 out]
                  }
                  frame 14 {
                    n1557 = property on="light_47" class="Bool (严格)"("Colors [4]"=w709) -> ()  [unwired: 2 in, 2 out]
                  }
                  frame 15 {
                    n1558 = property on="light_48" class="Bool (严格)"("Colors [4]"=w710) -> ()  [unwired: 2 in, 2 out]
                  }
                }
                n1559 = Replace Array Subset(array=w693, new element=w692, index (row)=w690, index (col)=2 ("索引 (列)")) -> (w691:string[][])
                n1560 = local write "D_IN_3"(w691) -> ()
              }
              frame 3 {
                n1561 = local read "D_IN_4"() -> (w715:string[][])
                n1562 = case shown="15" w712 {
                  tunnel: w711 -> [w717 w718 w719 w720 w721 w722 w723 w724 w725 w726 w727 w728 w729 w730 w731 w732]
                  frame 0, Default {
                    n1563 = property on="light_49" class="Bool (严格)"("Colors [4]"=w717) -> ()  [unwired: 2 in, 2 out]
                  }
                  frame 1 {
                    n1564 = property on="light_50" class="Bool (严格)"("Colors [4]"=w718) -> ()  [unwired: 2 in, 2 out]
                  }
                  frame 2 {
                    n1565 = property on="light_51" class="Bool (严格)"("Colors [4]"=w719) -> ()  [unwired: 2 in, 2 out]
                  }
                  frame 3 {
                    n1566 = property on="light_52" class="Bool (严格)"("Colors [4]"=w720) -> ()  [unwired: 2 in, 2 out]
                  }
                  frame 4 {
                    n1567 = property on="light_53" class="Bool (严格)"("Colors [4]"=w721) -> ()  [unwired: 2 in, 2 out]
                  }
                  frame 5 {
                    n1568 = property on="light_54" class="Bool (严格)"("Colors [4]"=w722) -> ()  [unwired: 2 in, 2 out]
                  }
                  frame 6 {
                    n1569 = property on="light_55" class="Bool (严格)"("Colors [4]"=w723) -> ()  [unwired: 2 in, 2 out]
                  }
                  frame 7 {
                    n1570 = property on="light_56" class="Bool (严格)"("Colors [4]"=w724) -> ()  [unwired: 2 in, 2 out]
                  }
                  frame 8 {
                    n1571 = property on="light_57" class="Bool (严格)"("Colors [4]"=w725) -> ()  [unwired: 2 in, 2 out]
                  }
                  frame 9 {
                    n1572 = property on="light_58" class="Bool (严格)"("Colors [4]"=w726) -> ()  [unwired: 2 in, 2 out]
                  }
                  frame 10 {
                    n1573 = property on="light_59" class="Bool (严格)"("Colors [4]"=w727) -> ()  [unwired: 2 in, 2 out]
                  }
                  frame 11 {
                    n1574 = property on="light_60" class="Bool (严格)"("Colors [4]"=w728) -> ()  [unwired: 2 in, 2 out]
                  }
                  frame 12 {
                    n1575 = property on="light_61" class="Bool (严格)"("Colors [4]"=w729) -> ()  [unwired: 2 in, 2 out]
                  }
                  frame 13 {
                    n1576 = property on="light_62" class="Bool (严格)"("Colors [4]"=w730) -> ()  [unwired: 2 in, 2 out]
                  }
                  frame 14 {
                    n1577 = property on="light_63" class="Bool (严格)"("Colors [4]"=w731) -> ()  [unwired: 2 in, 2 out]
                  }
                  frame 15 {
                    n1578 = property on="light_64" class="Bool (严格)"("Colors [4]"=w732) -> ()  [unwired: 2 in, 2 out]
                  }
                }
                n1579 = Replace Array Subset(array=w715, new element=w714, index (row)=w712, index (col)=2 ("索引 (列)")) -> (w713:string[][])
                n1580 = local write "D_IN_4"(w713) -> ()
              }
              frame 4 {
                n1581 = local read "D_IN_5"() -> (w737:string[][])
                n1582 = case shown="15" w734 {
                  tunnel: w733 -> [w739 w740 w741 w742 w743 w744 w745 w746 w747 w748 w749 w750 w751 w752 w753 w754]
                  frame 0, Default {
                    n1583 = property on="light_65" class="Bool (严格)"("Colors [4]"=w739) -> ()  [unwired: 2 in, 2 out]
                  }
                  frame 1 {
                    n1584 = property on="light_66" class="Bool (严格)"("Colors [4]"=w740) -> ()  [unwired: 2 in, 2 out]
                  }
                  frame 2 {
                    n1585 = property on="light_67" class="Bool (严格)"("Colors [4]"=w741) -> ()  [unwired: 2 in, 2 out]
                  }
                  frame 3 {
                    n1586 = property on="light_68" class="Bool (严格)"("Colors [4]"=w742) -> ()  [unwired: 2 in, 2 out]
                  }
                  frame 4 {
                    n1587 = property on="light_69" class="Bool (严格)"("Colors [4]"=w743) -> ()  [unwired: 2 in, 2 out]
                  }
                  frame 5 {
                    n1588 = property on="light_70" class="Bool (严格)"("Colors [4]"=w744) -> ()  [unwired: 2 in, 2 out]
                  }
                  frame 6 {
                    n1589 = property on="light_71" class="Bool (严格)"("Colors [4]"=w745) -> ()  [unwired: 2 in, 2 out]
                  }
                  frame 7 {
                    n1590 = property on="light_72" class="Bool (严格)"("Colors [4]"=w746) -> ()  [unwired: 2 in, 2 out]
                  }
                  frame 8 {
                    n1591 = property on="light_73" class="Bool (严格)"("Colors [4]"=w747) -> ()  [unwired: 2 in, 2 out]
                  }
                  frame 9 {
                    n1592 = property on="light_74" class="Bool (严格)"("Colors [4]"=w748) -> ()  [unwired: 2 in, 2 out]
                  }
                  frame 10 {
                    n1593 = property on="light_75" class="Bool (严格)"("Colors [4]"=w749) -> ()  [unwired: 2 in, 2 out]
                  }
                  frame 11 {
                    n1594 = property on="light_76" class="Bool (严格)"("Colors [4]"=w750) -> ()  [unwired: 2 in, 2 out]
                  }
                  frame 12 {
                    n1595 = property on="light_77" class="Bool (严格)"("Colors [4]"=w751) -> ()  [unwired: 2 in, 2 out]
                  }
                  frame 13 {
                    n1596 = property on="light_78" class="Bool (严格)"("Colors [4]"=w752) -> ()  [unwired: 2 in, 2 out]
                  }
                  frame 14 {
                    n1597 = property on="light_79" class="Bool (严格)"("Colors [4]"=w753) -> ()  [unwired: 2 in, 2 out]
                  }
                  frame 15 {
                    n1598 = property on="light_80" class="Bool (严格)"("Colors [4]"=w754) -> ()  [unwired: 2 in, 2 out]
                  }
                }
                n1599 = Replace Array Subset(array=w737, new element=w735, index (row)=w734, index (col)=2 ("索引 (列)")) -> (w736:string[][])
                n1600 = local write "D_IN_5"(w736) -> ()
              }
              frame 1 {
                n1601 = local read "D_IN_2"() -> (w759:string[][])
                n1602 = case shown="15" w756 {
                  tunnel: w755 -> [w761 w762 w763 w764 w765 w766 w767 w768 w769 w770 w771 w772 w773 w774 w775 w776]
                  frame 0, Default {
                    n1603 = property on="light_17" class="Bool (严格)"("Colors [4]"=w761) -> ()  [unwired: 2 in, 2 out]
                  }
                  frame 1 {
                    n1604 = property on="light_18" class="Bool (严格)"("Colors [4]"=w762) -> ()  [unwired: 2 in, 2 out]
                  }
                  frame 2 {
                    n1605 = property on="light_19" class="Bool (严格)"("Colors [4]"=w763) -> ()  [unwired: 2 in, 2 out]
                  }
                  frame 3 {
                    n1606 = property on="light_20" class="Bool (严格)"("Colors [4]"=w764) -> ()  [unwired: 2 in, 2 out]
                  }
                  frame 4 {
                    n1607 = property on="light_21" class="Bool (严格)"("Colors [4]"=w765) -> ()  [unwired: 2 in, 2 out]
                  }
                  frame 5 {
                    n1608 = property on="light_22" class="Bool (严格)"("Colors [4]"=w766) -> ()  [unwired: 2 in, 2 out]
                  }
                  frame 6 {
                    n1609 = property on="light_23" class="Bool (严格)"("Colors [4]"=w767) -> ()  [unwired: 2 in, 2 out]
                  }
                  frame 7 {
                    n1610 = property on="light_24" class="Bool (严格)"("Colors [4]"=w768) -> ()  [unwired: 2 in, 2 out]
                  }
                  frame 8 {
                    n1611 = property on="light_25" class="Bool (严格)"("Colors [4]"=w769) -> ()  [unwired: 2 in, 2 out]
                  }
                  frame 9 {
                    n1612 = property on="light_26" class="Bool (严格)"("Colors [4]"=w770) -> ()  [unwired: 2 in, 2 out]
                  }
                  frame 10 {
                    n1613 = property on="light_27" class="Bool (严格)"("Colors [4]"=w771) -> ()  [unwired: 2 in, 2 out]
                  }
                  frame 11 {
                    n1614 = property on="light_28" class="Bool (严格)"("Colors [4]"=w772) -> ()  [unwired: 2 in, 2 out]
                  }
                  frame 12 {
                    n1615 = property on="light_29" class="Bool (严格)"("Colors [4]"=w773) -> ()  [unwired: 2 in, 2 out]
                  }
                  frame 13 {
                    n1616 = property on="light_30" class="Bool (严格)"("Colors [4]"=w774) -> ()  [unwired: 2 in, 2 out]
                  }
                  frame 14 {
                    n1617 = property on="light_31" class="Bool (严格)"("Colors [4]"=w775) -> ()  [unwired: 2 in, 2 out]
                  }
                  frame 15 {
                    n1618 = property on="light_32" class="Bool (严格)"("Colors [4]"=w776) -> ()  [unwired: 2 in, 2 out]
                  }
                }
                n1619 = Replace Array Subset(array=w759, new element=w757, index (row)=w756, index (col)=2 ("索引 (列)")) -> (w758:string[][])
                n1620 = local write "D_IN_2"(w758) -> ()
              }
            }
          }
          frame #1 {
            n1621 = local write "同步_A1"(0 ("同步_A1")) -> ()
          }
        }
      }
    }
    n1622 = local read "关闭？"() -> (w634:bool)
  }
  n1623 = Release Notifier(notifier=w10, error in (no error)=w9) -> ()  [unwired: 1 in, 3 out]
